vi "Text control 2 v2.8.vi"() -> ()   [LabVIEW 2016]
panel:
  in  "Set Start Time":dbl caption="Set Start Time (s)"
  out "Total lines":i32
  out "Line running":i32
  in  "byte count":u32=64
  in  "Serial Settings:Serial End Mode for Reads":u16(ring)=2 items=["None", "LastBit", "TermChar"]
  in  "Timeout (ms)":u32=10000
  in  "Enable Termination\nChar (T)":bool=TRUE
  in  "Termination char\n(0xA = '\\n' = LF)\n(0xD = '\\r' = CR)":u8=13 format="%.0x"
  in  "flow control":u16(ring) items=["None"=0, "XON/XOFF"=1, "RTS/CTS"=2, "DTR/DSR"=4]
  in  "stop bits":u16(ring)=10 items=["1.0"=10, "1.5"=15, "2.0"=20]
  in  "parity":u16(ring) items=["None", "Odd", "Even", "Mark", "Space"]
  in  "data bits":u16=8 min=5 max=8 step=1
  in  "VISA resource name":refnum<visa-resource-name>="COM6"
  in  "baud rate":u32=9600
  out "Serial port output":string
  out "error out":errorcluster
  in  "Units":bool
  out "Elapsed Time":dbl caption="Elapsed Time (s)"
  out "Id max vs time":cluster{"Y data in":dbl[], "X data in":dbl[]}[](graph)
  out "Ig":dbl format="%.2e"
  out "Id":dbl format="%.2e"
  out "Is":dbl format="%.2e"
  out "I vs Vg":cluster{"Y data in":dbl[], "X data in":dbl[]}[](graph)
  in  "Panel Controls 2":T1={"Emergency Stop"=refnum, "TransGraph Max"=1e-05, "Text/Graph (text=false)"=TRUE, "TransGraph Min"=1e-11} {"TransGraph Min" format="%.2e"; "TransGraph Max" format="%.2e"}
  out "Command running:":string="#output s 0 0 0 -0.008 0.008 0.002"
  in  "Standby":T2
  in  "Full Reset":bool
  in  "SMU4":cluster{"on/off":bool, "Voltage":dbl} {"Voltage" min=-100.0 max=100.0 format="%.2f"}
  in  "Source/Drain Range":u8(slide)=6 max=11 scale=0.0..11.0
  in  "Source/Drain\nRange mode":u16(ring) items=["Auto", "Limited", "Fixed"]
  in  "Gate Range":u8(slide)=6 max=11 scale=0.0..11.0
  in  "Gate Range\nmode":u16(ring) items=["Auto", "Limited", "Fixed"]
  in  "Gate":T3={"Gate Start"=0.0, "Gate Stop"=2.0, "Gate Step (linear only)"=1.0, "Gate Compliance"=0.0001, "Gate PComp"=0.0, "Range mode"=0, "Range"=6} {"Range" max=11 scale=0.0..11.0; "Range mode" items=["Auto", "Limited", "Fixed"]; "Gate PComp" format="%^.2e"; "Gate Compliance" format="%^.2e"; "Gate Step (linear only)" format="%^.4e"; "Gate Stop" format="%^.4e"; "Gate Start" format="%^.4e"}
  in  "Drain 2":T4={"Drain Start"=0.0, "Drain Stop"=2.0, "Drain Compliance"=0.0001, "Drain Step"=1.0, "Drain PComp"=0.0, "Range mode"=0, "Range"=6} {"Range" max=11 scale=0.0..11.0; "Range mode" items=["Auto", "Limited", "Fixed"]; "Drain PComp" format="%^.2e"; "Drain Step" format="%^.4e"; "Drain Compliance" format="%^.2e"; "Drain Stop" format="%^.4e"; "Drain Start" format="%^.4e"}
  in  "Timings 2":T5={"integration time"=0, "Short/Long integration time"=0.00064, "hold time (sec)"=0.0, "delay time (sec)"=0.0, "Step Time (0 disables)"=0.0, "sweep method"=0, "Pulse period"=0.005, "Base voltage"=0.0, "Pulse width"=0.0005} {"Pulse width" min=0.0005 max=0.1 step=0.0001 format="%.4f"; "Base voltage" format="%^.4e"; "Pulse period" min=0.005 max=1.0 step=0.0001 format="%.4f"; "sweep method" items=["Continuous", "Pulsed"]; "Step Time (0 disables)" format="%.2f"; "delay time (sec)" format="%.4f"; "hold time (sec)" format="%.4f"; "Short/Long integration time" format="%^.0e"; "integration time" scale=0.0..2.0}
  in  "Panel Controls":T6={"Emergency Stop"=refnum, "TransGraph Max"=1e-05, "Text/Graph (text=false)"=TRUE} {"TransGraph Max" format="%.2e"}
  in  "Interrupt run":bool
  in  "Drain: Compliance":dbl=0.001 format="%.8f"
  in  "Gate: Compliance":dbl=0.001 format="%.8f"
  out "Path":path=path "C:/users/rlp38/09Apr2009LTtesting/test2.txt"
  in  "hold time /s":dbl format="%.2f"
  in  "delay time /s":dbl format="%.2f"
  in  "integration time":u32(slide) max=2 step=1 scale=0.0..2.0
  in  "Integration time (short)":dbl=0.0019 min=8e-05 max=0.0019 step=8e-05 format="%^.0e"
  in  "Integration time (long)":dbl=0.32 min=0.04 max=2.0 step=0.02 format="%.2f"
  in  "Step delay /s":dbl format="%.2f"
  in  "Program":string="#pulsedstressV d 0.03 20 0 0.5 0.0827 5\n#\n#itime s\n#gaterangemode l\n#drainrangemode l\n#pulsed on 0.05 0 0.02\n#transfer d 1 -1 -0.1 -1 -1 0\n#wait-min 1\n#transfer d 1 -1 -0.1 -1 -1 0\n#output d 0 -1 -0.5 0 -1 -0.1\n#transfer d -10 40 1 5 40 35\n#transfer d -10 40 1 5 40 35\n#output d 0 40 20 0 40 1\n#\n#\n#sample 1 0.008 221 6 0.003\n#samplei 400e-6 200 6 0.002 0.1\n#vsu2pulse -10 4\n#\n#stressV 0.016 0.03 2e-4 0.1e-3 11\n#stressI 220e-7 0.08 15\n#transfer s -1 1 0.5 -0.005 0.005 0.005\n#output s 0 0 0 -0.008 0.008 0.002\n"
  # "Serial port settings"
  # "Time"
  # "Sec"
  # "Min"
  # "100 samples is approx 13s with medium integration"
  # "Syntax:\nitime [s|m|l]\ngaterangemode [a|l|f]\ndrainrangemode [a|l|f]\npulsed [on|off] PulsePeriod(sec) PulseBaseVoltage PulseONWidth(sec)\nstandby [on l off]\nwait NumMilliseconds\nwait-min NumMinutes\n# texthere = comment\ntransfer [s|d] VgStart VgStop VgStep VdStart VdStop VdStep\noutput [s|d] VgStart VgStop VgStep VdStart VdStop VdStep\nsample Vg Vd NumSamples Time(s) SampleInterval(s)\nsamplei Idg NumSamples Time(s) SampleInterval(s) VDGcompliance\n# if in doubt use SampleInterval(s) = 0.004\nstressV VG VD IGcompliance IDcompliance Duration(sec)\nstressI IDG VDGcompliance Duration(sec)\nvsu2pulse Bias Duration(s)\npulsedstressV [s|d] VEstop VgON VgOFF Period(s) PulseONwidth(s) Vd\nsample-fpp Vg Vd NumSamples Time\nresample-fpp Vg Vd\ntransfer-fpp [s|d] VgStart VgStop VgStep VdStart VdStop VdStep\noutput-fpp [s|d] VgStart VgStop VgStep VdStart VdStop VdStep\nserial SerialPortCommand"
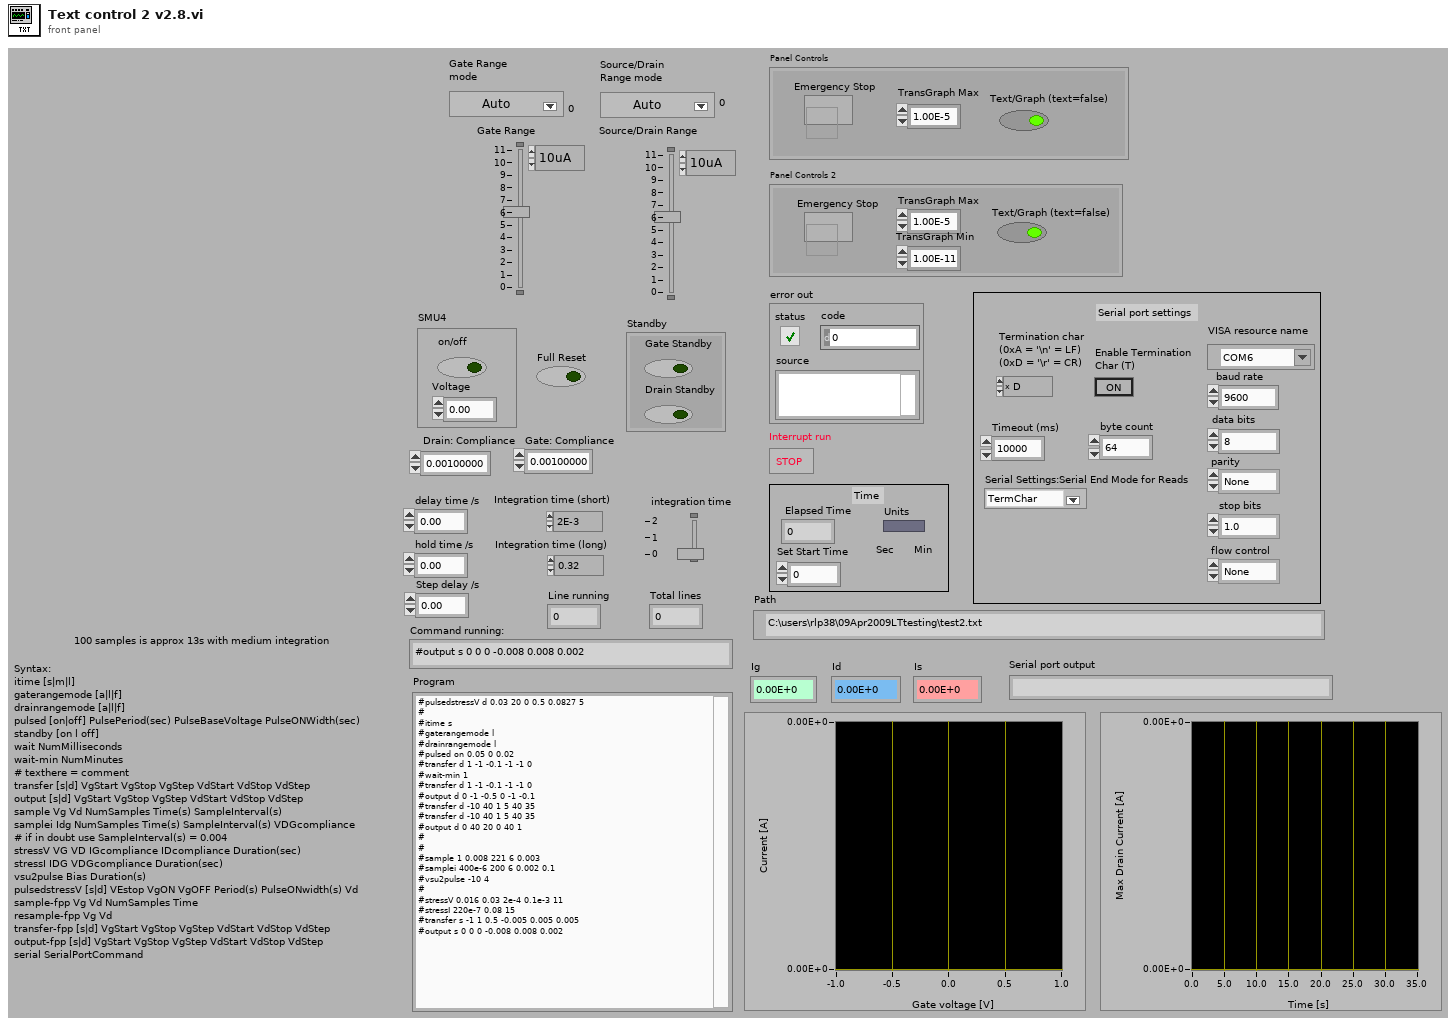
[diagram p1: front panel]
types:
  T1 = cluster{"Emergency Stop":refnum<vi>, "TransGraph Max":dbl, "Text/Graph (text=false)":bool, "TransGraph Min":dbl}
  T2 = cluster{"Gate Standby":bool, "Drain Standby":bool}
  T3 = cluster{"Gate Start":dbl, "Gate Stop":dbl, "Gate Step (linear only)":dbl, "Gate Compliance":dbl, "Gate PComp":dbl, "Range mode":u16, "Range":u8}
  T4 = cluster{"Drain Start":dbl, "Drain Stop":dbl, "Drain Compliance":dbl, "Drain Step":dbl, "Drain PComp":dbl, "Range mode":u16, "Range":u8}
  T5 = cluster{"integration time":u32, "Short/Long integration time":dbl, "hold time (sec)":dbl, "delay time (sec)":dbl, "Step Time (0 disables)":dbl, "sweep method":u16, "Pulse period":dbl, "Base voltage":dbl, "Pulse width":dbl}
  T6 = cluster{"Emergency Stop":refnum<vi>, "TransGraph Max":dbl, "Text/Graph (text=false)":bool}
  T7 = enum16{"open", "replace", "create", "open or create", "replace or create", "replace or create with confirmation"}
  T8 = cluster{"V2 Start":dbl, "V2 Step":dbl, "Number of points":i32}
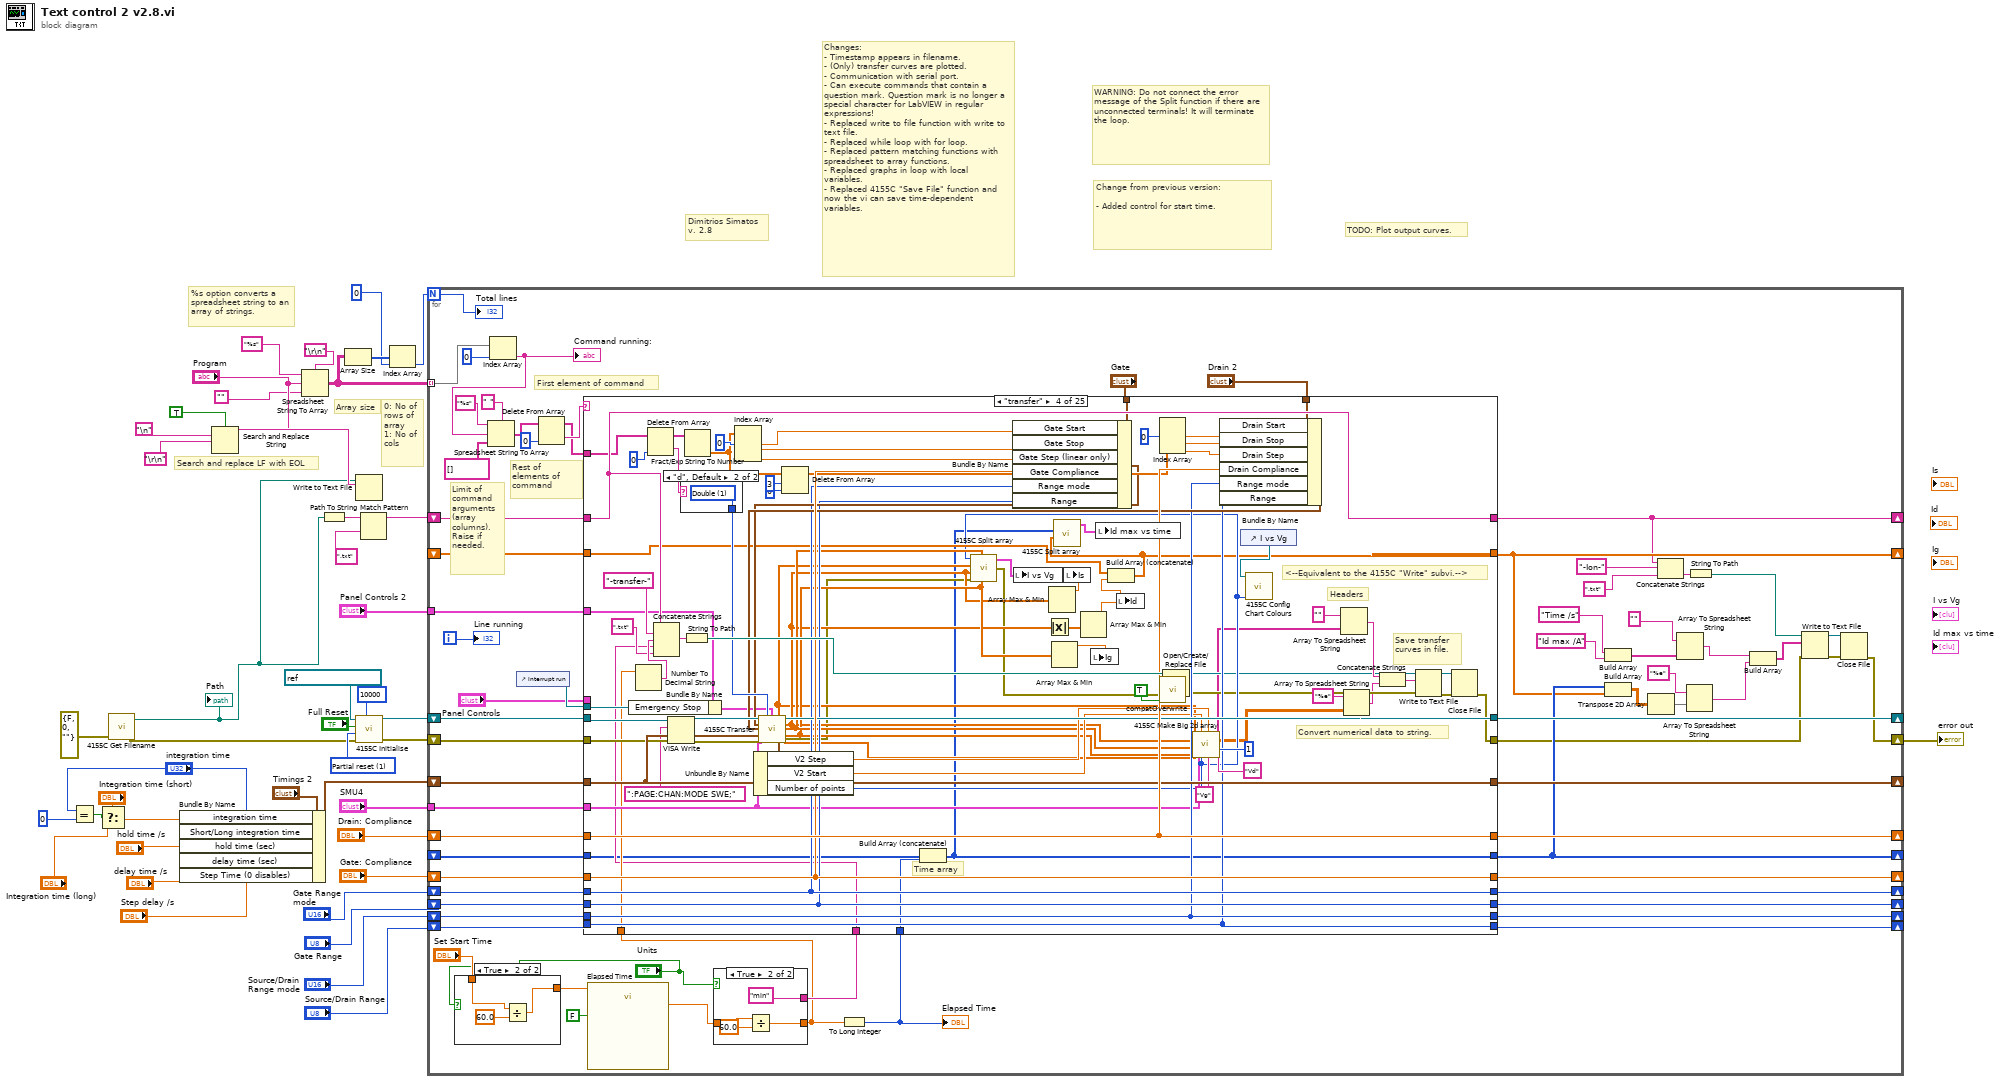
[diagram p0: block diagram]
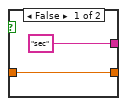
[diagram p3: hidden frame]
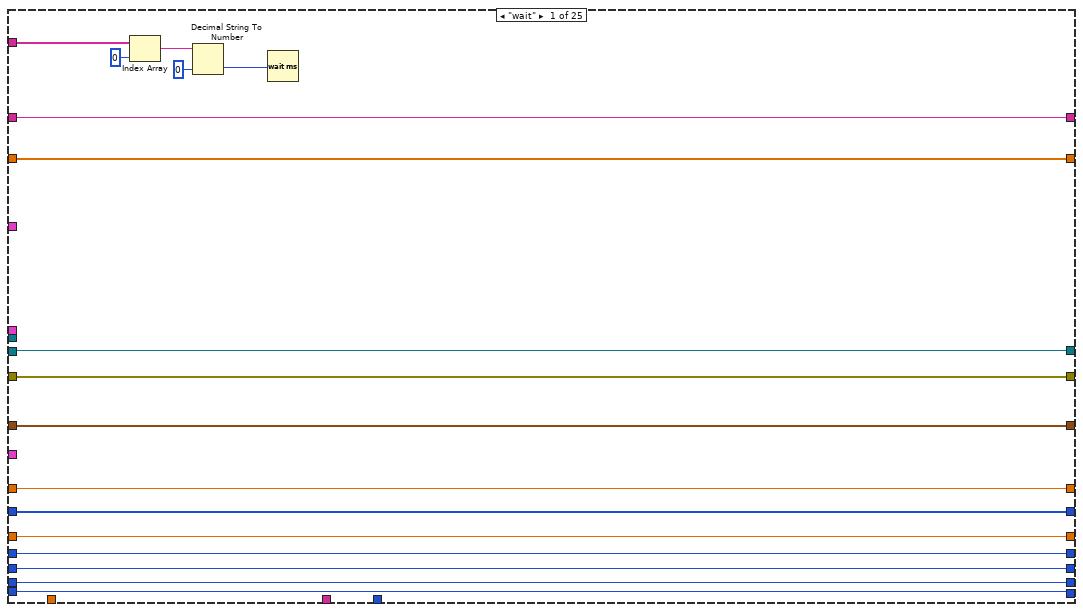
[diagram p4: hidden frame]
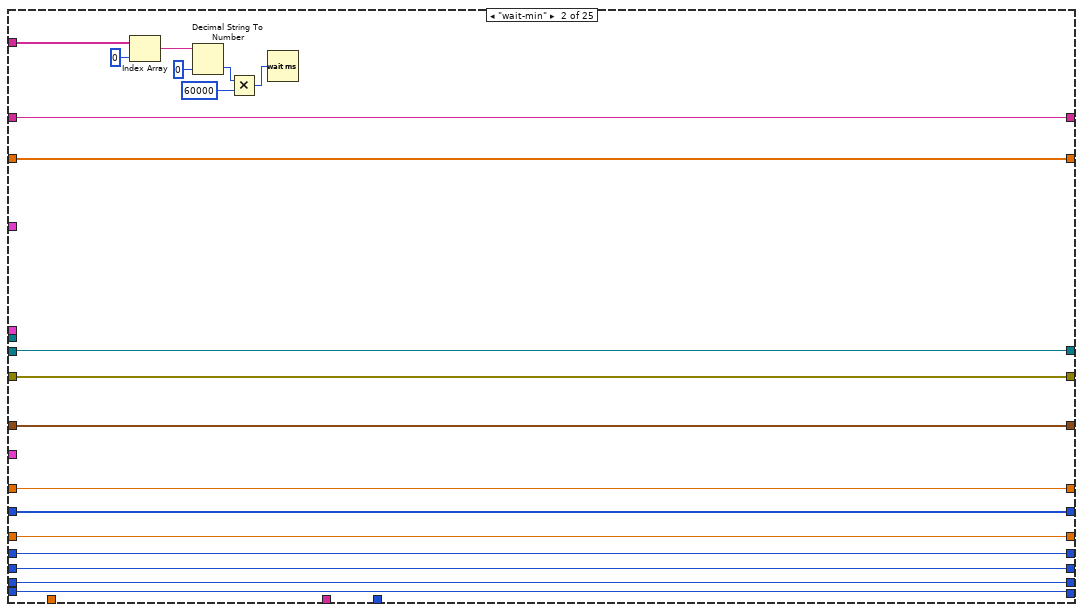
[diagram p5: hidden frame]
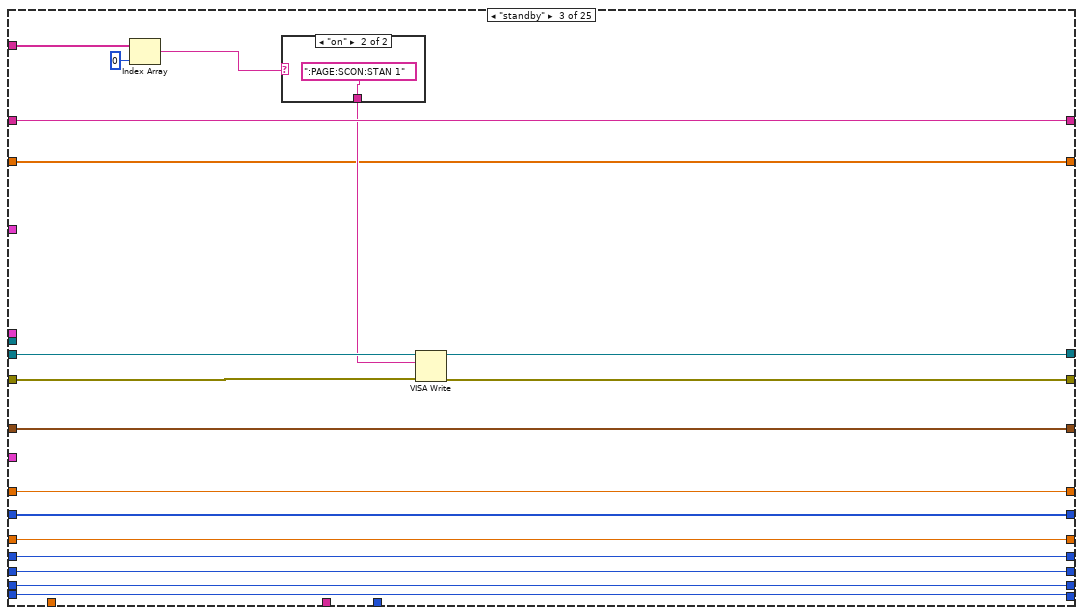
[diagram p6: hidden frame]
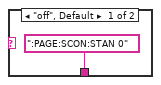
[diagram p7: hidden frame]
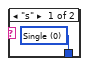
[diagram p8: hidden frame]
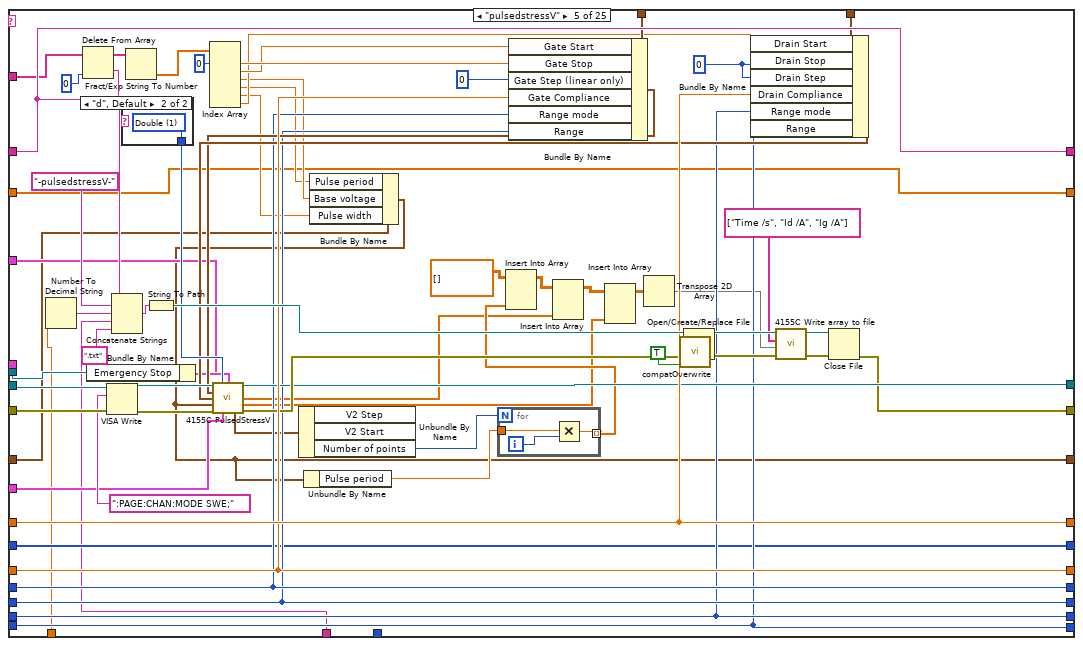
[diagram p9: hidden frame]
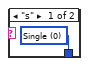
[diagram p10: hidden frame]
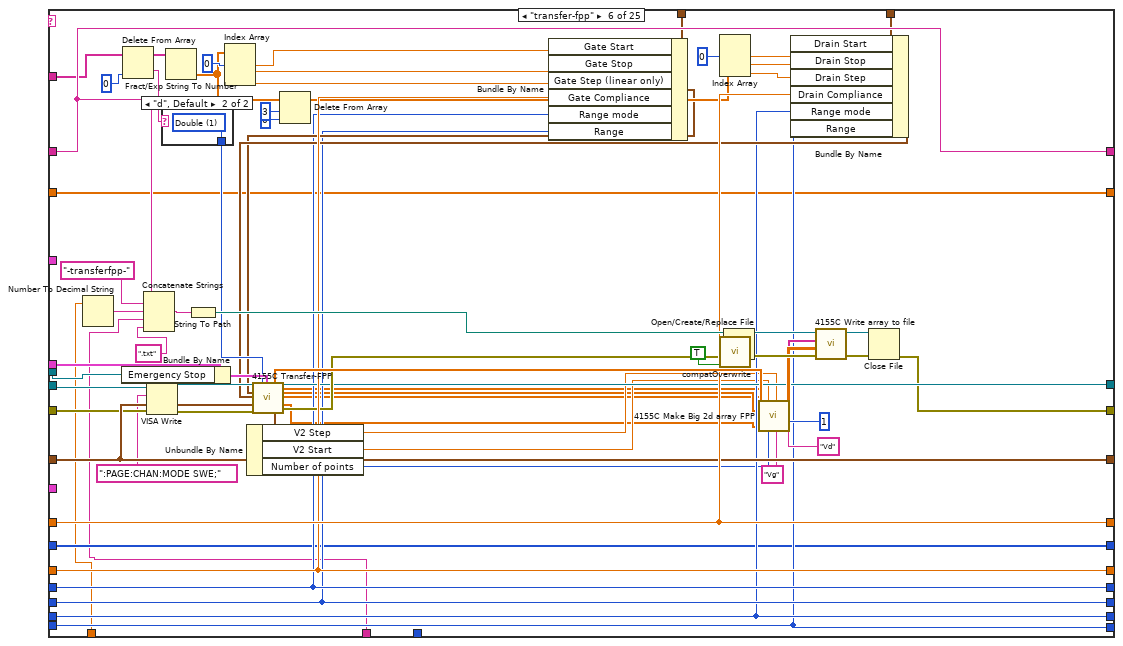
[diagram p11: hidden frame]
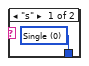
[diagram p12: hidden frame]
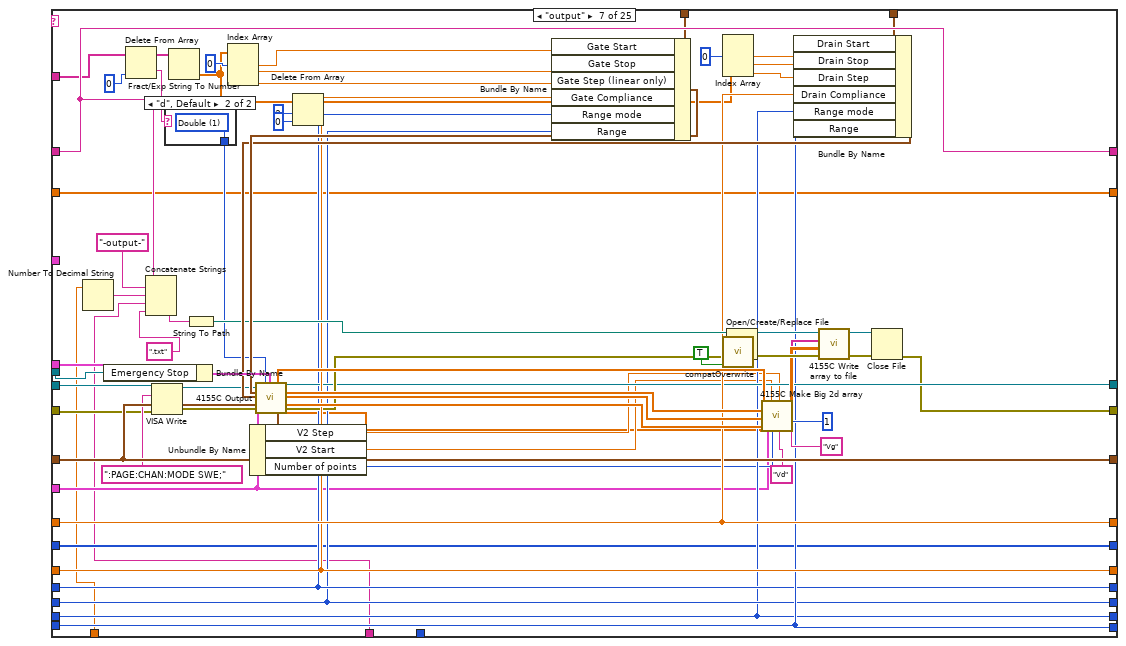
[diagram p13: hidden frame]
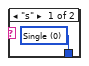
[diagram p14: hidden frame]
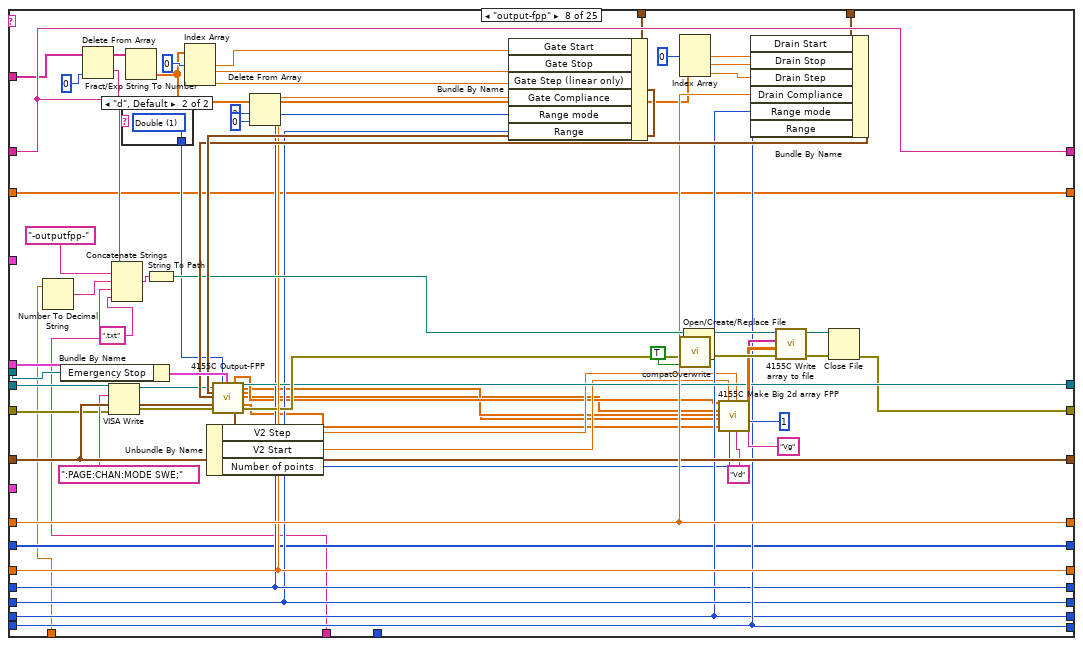
[diagram p15: hidden frame]
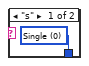
[diagram p16: hidden frame]
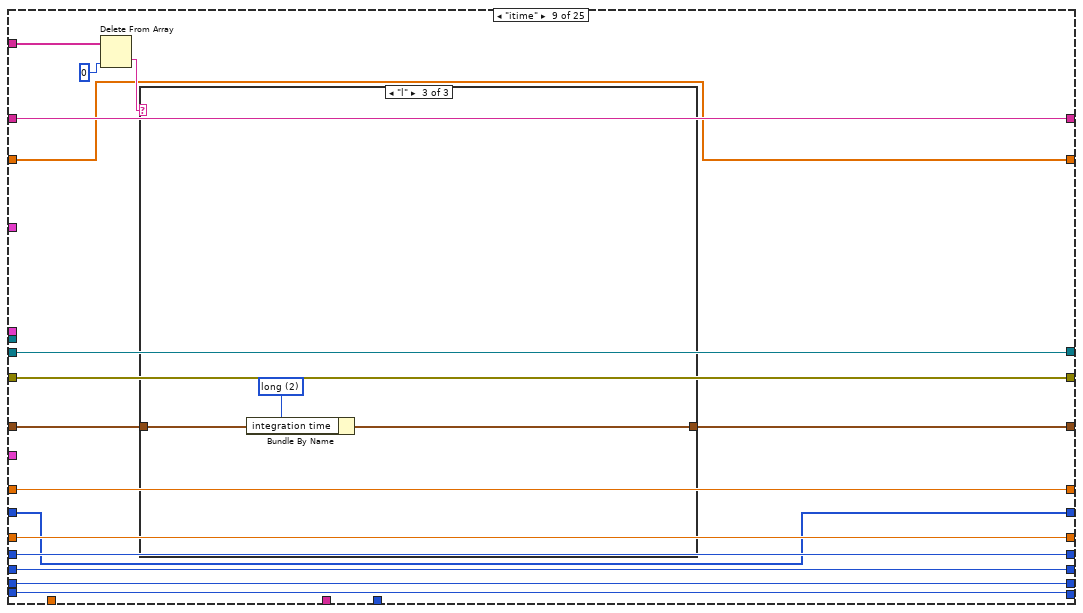
[diagram p17: hidden frame]
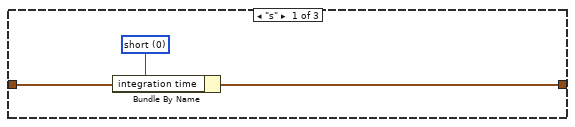
[diagram p18: hidden frame]
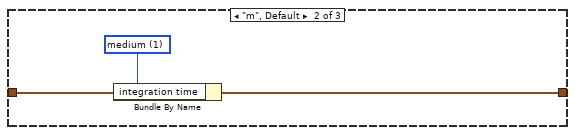
[diagram p19: hidden frame]
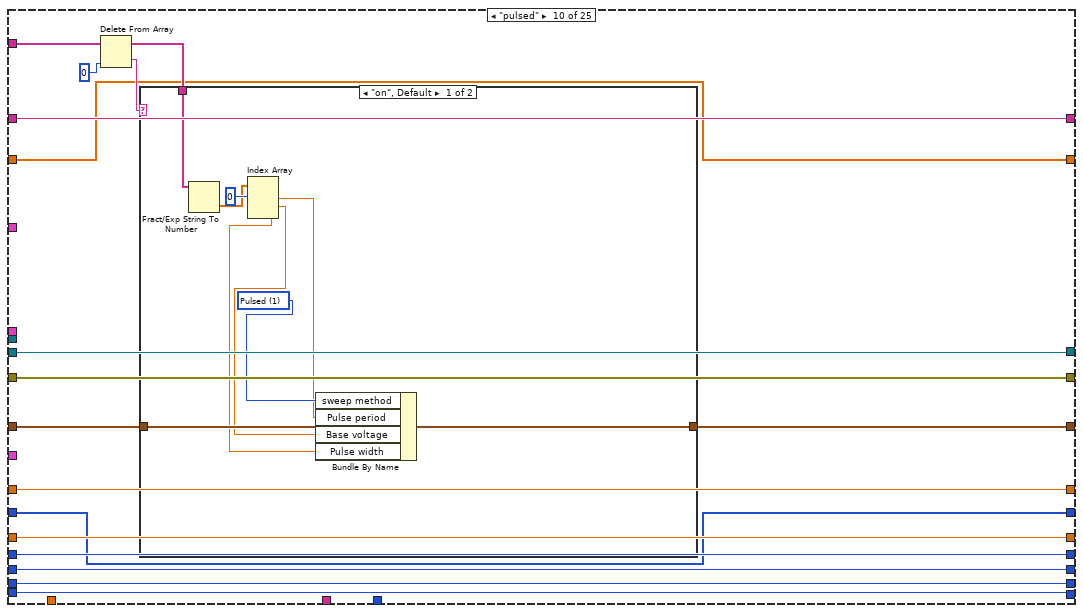
[diagram p20: hidden frame]
diagram:
  w35 = u16 1 items=["Reset All", "Partial reset"] ("Type of reset")
  # "TODO: Plot output curves."
  # "WARNING: Do not connect the error message of the Split function if there are unconnected terminals! It will terminate the loop."
  # "Array size"
  # "%s option converts a spreadsheet string to an array of strings."
  # "0: No of rows of array\n1: No of cols"
  # "Change from previous version:\n\n- Added control for start time."
  # "Dimitrios Simatos\nv. 2.8"
  # "Changes:\n- Timestamp appears in filename.\n- (Only) transfer curves are plotted.\n- Communication with serial port.\n- Can execute commands that contain a question mark. Question mark is no longer a special character for LabVIEW in regular expressions!\n- Replaced write to file function with write to text file.\n- Replaced while loop with for loop.\n- Replaced pattern matching functions with spreadsheet to array functions.\n- Replaced graphs in loop with local variables.\n- Replaced 4155C \"Save File\" function and now the vi can save time-dependent variables."
  # "Search and replace LF with EOL"
  n1 = Equal?(x="integration time", y=u32 0) -> (x = y?=w39:bool)
  n2 = Select(t="Integration time (short)", s=w39, f="Integration time (long)") -> (s? t:f=w43:dbl)
  n3 = call "4155C Get Filename.vi"("error in (no error)"=errorcluster {"status"=FALSE, "code"=0, "source"=""}) -> ("error out"=w30:errorcluster, "path"=w2:path)  [unwired: 2 in, 1 out]
  "Path" <- w2
  n4 = Bundle By Name(cluster="Timings 2", "integration time"="integration time", "Short/Long integration time"=w43, "hold time (sec)"="hold time /s", "delay time (sec)"="delay time /s", "Step Time (0 disables)"="Step delay /s") -> (w27:T5)
  n5 = Search and Replace String(replace all?=TRUE ("replace all? (F)"), input string="Program", search string="\n", replace string="\r\n") -> (result string=w17:string)  [unwired: 4 in, 3 out]
  n6 = Spreadsheet String To Array(delimiter (Tab)="\r\n", format string="%s", spreadsheet string="Program", array type (2D Dbl)="") -> (array=w8:string[][])
  n7 = Path To String(path=w2) -> (string=w5:string)
  n8 = Array Size(array=w8) -> (size(s)=w12:i32[])
  n9 = Write to Text File(file (use dialog)=w2, text=w17) -> ()  [unwired: 2 in, 3 out]
  n10 = call "4155C Initialise.vi"("VISA resource name in"=refnum<visa-resource-name> "GPIB0::14::INSTR", "Reset"="Full Reset", "Type of reset"=w35, "error in (no error)"=w30, "VISA Timeout Value"=u32 10000) -> ("VISA Resource Name out"=w29:refnum<visa-resource-name>, "error out"=w28:errorcluster)
  n11 = Match Pattern(string=w5, regular expression=".txt") -> (before substring=w3:string)  [unwired: 1 in, 3 out]
  n12 = Index Array(array=w12, index=0) -> (element=w10:i32)
  n13 = for {
    N: w10 -> [w77]
    tunnel: "SMU4" -> [w89]
    shift-left: "Source/Drain Range" -> [w94]
    shift-right: [w90] -> _
    shift-left: "Source/Drain\nRange mode" -> [w95]
    shift-right: [w91] -> _
    shift-left: "Gate Range" -> [w96]
    shift-right: [w92] -> _
    shift-left: "Gate Range\nmode" -> [w97]
    shift-right: [w93] -> _
    shift-left: "Gate: Compliance" -> [w106]
    shift-right: [w102] -> _
    shift-left: "Drain: Compliance" -> [w107]
    shift-right: [w103] -> _
    shift-left: w27 -> [w108]
    shift-right: [w104] -> _
    shift-left: w28 -> [w109]
    shift-right: [w45] -> w1
    shift-left: w29 -> [w110]
    shift-right: [w105] -> _
    shift-left: w3 -> [w111]
    shift-right: [w50] -> _
    tunnel: "Panel Controls 2" -> [w88]
    shift-right: [w53] -> _
    shift-left: _ -> [w87]
    shift-right: [w54] -> _
    shift-left: _ -> [w83]
    tunnel: w8 -> [w80] mode=indexing
    i -> [w78]
    # "Limit of command arguments (array columns). Raise if needed."
    # "Rest of elements of command"
    # "First element of command"
    n14 = case shown="True" "Units" {
      tunnel: "Set Start Time" -> [w112 w114]
      tunnel: [w112 w113] -> w48
      frame False {
      }
      frame True {
        n15 = Divide(x=w114, y=60.0) -> (x/y=w113:dbl)
      }
    }
    n16 = Index Array(array=w80, index=0 ("line index")) -> (element=w73:string)
    "Command running:" <- w73
    n17 = Spreadsheet String To Array(delimiter (Tab)=" ", format string="%s", spreadsheet string=w73, array type (2D Dbl)=string[] []) -> (array=w70:string[])
    n18 = control-ref of="Interrupt run"() -> (w101:refnum<vi>)
    n19 = Delete From Array(array=w70, index=0) -> (deleted portion=w71:string, array with subset deleted=w69:string[])  [unwired: 1 in]
    n20 = call "Elapsed Time"("Time Target (s)"=w48, "Auto Reset"=FALSE) -> ("Elapsed Time (s)"=w84:dbl)  [unwired: 10 in, 7 out]
    n21 = case shown="True" "Units" {
      tunnel: ["sec" "min"] -> w85
      tunnel: [w116 w120] -> w82
      tunnel: w84 -> [w116 w119]
      frame False {
      }
      frame True {
        n22 = Divide(x=w119, y=60.0) -> (x/y=w120:dbl)
      }
    }
    n23 = To Long Integer(number=w82) -> (32bit integer=w81:i32)
    "Elapsed Time" <- w81
    n24 = case shown="\"transfer\"" w71 {
      tunnel: w69 -> [w138 w157 w175 w252 w316 w385 w452 w527 w565 w591 w618 w643 w664 w678 _ _ w782 w843 _ w908 w952 w994 w1064 w1126 w1133]
      tunnel: w111 -> [w133 w153 w173 w259 w323 w393 w460 w535 w554 w580 w610 w636 w658 w671 w690 w732 w760 w825 w856 w895 w939 w982 w1058 w1122 w1135]
      tunnel: w110 -> [w132 w152 w164 w230 w307 w362 w428 w503 w555 w581 w611 w637 w659 w672 w695 w734 w788 w849 w860 w914 w958 w1000 w1070 w1080 w1139]
      tunnel: w109 -> [w131 w151 w163 w229 w306 w361 w425 w500 w556 w582 w612 w638 w660 w673 w694 w705 w787 w848 w859 w913 w957 w999 w1069 w1079 w1138]
      tunnel: w108 -> [w130 w150 w172 w255 w282 w389 w456 w531 w564 w590 w609 w635 w657 w670 w693 w729 w751 w817 w865 w888 w932 w975 w1057 w1121 w1140]
      tunnel: w107 -> [w129 w149 w171 w257 w321 w391 w458 w533 w563 w589 w617 w642 w663 w677 w692 w714 w786 w847 w868 w912 w956 w998 w1068 w1130 w1141]
      tunnel: w106 -> [w128 w148 w170 w256 w320 w390 w457 w532 w562 w588 w616 w641 w662 w676 w691 w715 w761 w826 w867 w896 w940 w983 w1059 w1123 w1143]
      tunnel: [w132 w152 w162 w254 w318 w387 w454 w529 w555 w581 w611 w637 w659 w672 w695 w734 w752 w799 w858 w889 w933 w976 w1010 w1082 w1139] -> w105
      tunnel: [w131 w151 w161 w253 w317 w386 w453 w528 w556 w582 w612 w638 w660 w673 w694 w704 w762 w800 w857 w897 w941 w984 w1009 w1081 w1137] -> w46
      tunnel: [w130 w150 w172 w255 w278 w389 w456 w531 w557 w583 w609 w635 w657 w670 w693 w729 w751 w817 w865 w888 w932 w975 w1057 w1121 w1140] -> w104
      tunnel: [w129 w149 w171 w257 w321 w391 w458 w533 w563 w589 w617 w642 w663 w677 w692 w714 w786 w847 w868 w912 w956 w998 w1068 w1130 w1141] -> w103
      tunnel: [w128 w148 w170 w256 w320 w390 w457 w532 w562 w588 w616 w641 w662 w676 w691 w715 w761 w826 w867 w896 w940 w983 w1059 w1123 w1143] -> w102
      tunnel: [w133 w153 w173 w259 w323 w393 w460 w535 w554 w580 w610 w636 w658 w671 w690 w732 w760 w825 w856 w895 w939 w982 w1058 w1122 w1135] -> w50
      tunnel: w101 -> [_ _ _ w262 w327 w398 w468 w539 _ _ _ _ _ _ _ _ w757 w822 _ w894 w938 w981 w1030 w1098 _]
      tunnel: "Gate" -> [_ _ _ w239 w310 w372 w439 w514 _ _ _ _ _ _ _ _ _ _ _ _ _ _ _ _ _]
      tunnel: "Drain 2" -> [_ _ _ w238 w309 w371 w438 w513 _ _ _ _ _ _ _ _ _ _ _ _ _ _ _ _ _]
      tunnel: "Panel Controls" -> [_ _ _ _ _ w370 w437 w512 _ _ _ _ _ _ _ _ _ _ _ _ _ _ _ _ _]
      tunnel: w97 -> [w127 w147 w169 w223 w300 w355 w423 w498 w561 w587 _ w634 w656 w669 w689 w716 w747 w813 w861 w884 w928 w971 w1053 w1117 w1144]
      tunnel: w96 -> [w126 w146 w168 w222 w299 w354 w422 w497 w560 w586 w615 _ w647 w675 w688 w717 w748 w814 w862 w885 w929 w972 w1054 w1118 w1145]
      tunnel: w95 -> [w125 w145 w167 w221 w298 w353 w421 w496 w559 w585 w614 w640 w661 _ w687 w718 w749 w815 w863 w886 w930 w973 w1055 w1119 w1146]
      tunnel: w94 -> [w124 w144 w166 w220 w297 w352 w424 w499 w558 w584 w613 w639 _ w674 w686 w719 w750 w816 w864 w887 w931 w974 w1056 w1120 w1147]
      tunnel: [w127 w147 w169 w223 w300 w355 w423 w498 w561 w587 w608 w634 w656 w669 w689 w716 w747 w813 w861 w884 w928 w971 w1053 w1117 w1144] -> w93
      tunnel: [w126 w146 w168 w222 w299 w354 w422 w497 w560 w586 w615 w626 w647 w675 w688 w717 w748 w814 w862 w885 w929 w972 w1054 w1118 w1145] -> w92
      tunnel: [w125 w145 w167 w221 w298 w353 w421 w496 w559 w585 w614 w640 w661 w668 w687 w718 w749 w815 w863 w886 w930 w973 w1055 w1119 w1146] -> w91
      tunnel: [w124 w144 w166 w220 w297 w352 w424 w499 w558 w584 w613 w639 w648 w674 w686 w719 w750 w816 w864 w887 w931 w974 w1056 w1120 w1147] -> w90
      tunnel: w89 -> [_ _ _ w215 w294 _ w416 _ _ _ _ _ _ _ _ _ _ _ _ _ _ _ _ _ _]
      tunnel: w88 -> [_ _ _ w213 w293 _ _ _ _ _ _ _ _ _ _ _ _ _ _ _ _ _ _ _ _]
      tunnel: [w123 w140 w159 w181 w270 w342 w413 w485 w553 w578 w607 w625 w646 w667 w685 w700 w739 w797 w855 w873 w921 w965 w1007 w1075 w1136] -> w53
      tunnel: w87 -> [w123 w140 w159 w204 w270 w342 w413 w485 w553 w578 w607 w625 w646 w667 w685 w700 w739 w797 w855 w873 w921 w965 w1007 w1075 w1136]
      tunnel: w82 -> [_ _ _ w200 w267 w340 w410 w482 _ _ _ _ _ _ _ w698 w737 w794 _ w870 w918 w962 w1004 w1071 _]
      tunnel: w85 -> [_ _ _ w197 w266 w338 w409 w481 _ _ _ _ _ _ _ w696 w735 w793 _ w869 w917 w961 w1003 w1072 _]
      tunnel: w81 -> [_ _ _ w182 _ _ _ _ _ _ _ _ _ _ _ _ _ _ _ _ _ _ _ _ _]
      tunnel: [w122 w139 w158 w180 w269 w341 w412 w484 w552 w577 w606 w624 w645 w666 w684 w699 w738 w796 w854 w872 w920 w964 w1006 w1074 w1142] -> w54
      tunnel: w83 -> [w122 w139 w158 w196 w269 w341 w412 w484 w552 w577 w606 w624 w645 w666 w684 w699 w738 w796 w854 w872 w920 w964 w1006 w1074 w1142]
      frame "wait" {
        n25 = Index Array(array=w138, index=0 ("Index")) -> (element=w136:string)
        n26 = Decimal String To Number(string=w136, default (0L)=u32 0) -> (number=w135:u32)  [unwired: 1 in, 1 out]
        n27 = Wait (ms)(milliseconds to wait=w135) -> ()  [unwired: 1 out]
      }
      frame "wait-min" {
        n28 = Index Array(array=w157, index=0 ("Index")) -> (element=w155:string)
        n29 = Decimal String To Number(string=w155, default (0L)=u32 0) -> (number=w143:u32)  [unwired: 1 in, 1 out]
        n30 = Multiply(x=w143, y=u32 60000) -> (x*y=w142:u32)
        n31 = Wait (ms)(milliseconds to wait=w142) -> ()  [unwired: 1 out]
      }
      frame "standby" {
        n32 = Index Array(array=w175, index=0 ("Index")) -> (element=w165:string)
        n33 = case shown="\"on\"" w165 {
          tunnel: [":PAGE:SCON:STAN 0" ":PAGE:SCON:STAN 1"] -> w160
          frame "off", Default {
          }
          frame "on" {
          }
        }
        n34 = VISA Write(VISA resource name=w164, write buffer=w160, error in (no error)=w163) -> (VISA resource name out=w162:refnum<visa-resource-name>, error out=w161:errorcluster)  [unwired: 1 out]
      }
      frame "transfer" {
        # "<--Equivalent to the 4155C \"Write\" subvi.-->"
        # "Headers"
        # "Convert numerical data to string."
        # "Save transfer curves in file."
        # "Time array"
        n35 = Bundle By Name(cluster=w213, "Emergency Stop"=w262) -> (w214:T1)
        n36 = Number To Decimal String(number=w200) -> (decimal integer string=w199:string)  [unwired: 1 in]
        n37 = Delete From Array(array=w252, index=0 ("Index")) -> (deleted portion=w250:string, array with subset deleted=w249:string[])  [unwired: 1 in]
        n38 = Concatenate Strings(w259, "-transfer-" ("Prefix"), w199, w197, ".txt" ("Suffix")) -> (w261:string)
        n39 = VISA Write(VISA resource name=w230, write buffer=":PAGE:CHAN:MODE SWE;" ("write buffer (\"\")"), error in (no error)=w229) -> (VISA resource name out=w227:refnum<visa-resource-name>, error out=w228:errorcluster)  [unwired: 1 out]
        n40 = case shown="\"d\", Default" w250 {
          tunnel: [w264 w265] -> w248
          frame "s" {
            w264 = u16 0 items=["Single", "Double"] ("sweep mode")
          }
          frame "d", Default {
            w265 = u16 1 items=["Single", "Double"] ("sweep mode")
          }
        }
        n41 = String To Path(string=w261) -> (path=w258:path)
        n42 = Fract/Exp String To Number(string=w249) -> (number=w234:dbl[])  [unwired: 3 in, 1 out]
        n43 = Index Array(array=w234, index #1=0 ("Index")) -> (element #1=w247:dbl, element #2=w246:dbl, element #3=w245:dbl)  [unwired: 2 in]
        n44 = Delete From Array(array=w234, length=3 ("Length"), index=0 ("Index")) -> (array with subset deleted=w232:dbl[])  [unwired: 1 out]
        n45 = Build Array (concatenate)(w196, w182) -> (w180:i32[])
        n46 = Bundle By Name(cluster=w239, "Gate Start"=w247, "Gate Stop"=w246, "Gate Step (linear only)"=w245, "Gate Compliance"=w256, "Range mode"=w223, "Range"=w222) -> (w224:T3)
        n47 = Index Array(array=w232, index #1=0 ("Index")) -> (element #1=w242:dbl, element #2=w241:dbl, element #3=w240:dbl)  [unwired: 2 in]
        n48 = call <vilib>:"compatOverwrite.vi"("overwrite (F)"=TRUE) -> ("overwrite?"=w212:T7)
        n49 = Bundle By Name(cluster=w238, "Drain Start"=w242, "Drain Stop"=w241, "Drain Step"=w240, "Drain Compliance"=w257, "Range mode"=w221, "Range"=w220) -> (w225:T4)
        n50 = call "4155C Transfer.vi"("VISA resource name in"=w227, "Gate"=w224, "Drain"=w225, "Timings"=w255, "error in (no error)"=w228, "SMU4"=w215, "sweep mode"=w248, "Panel Controls"=w214) -> ("VG"=w205:dbl[], "Outparams"=w219:T8, "VISA Resource Name out"=w254:refnum<visa-resource-name>, "IS"=w206:dbl[], "ID"=w211:dbl[], "IG"=w207:dbl[], "error out"=w192:errorcluster, "SMU4"=w216:dbl[])  [unwired: 12 in]
        n51 = Unbundle By Name(w219) -> ("V2 Step"=w218:dbl, "V2 Start"=w217:dbl, "Number of points"=w202:i32)
        n52 = call "4155C Split array.vi"("Number of VAR2 steps"=w202, "Y2 data in"=w211, "X data in"=w205, "Y1 data in"=w206, "Y3 data in"=w207, "error in (no error)"=w192) -> ("Array of clusters"=w195:cluster{"Y data in":dbl[], "X data in":dbl[]}[], "error out"=w193:errorcluster)  [unwired: 1 in]
        n53 = local write "I vs Vg"(w195) -> ()
        n54 = Absolute Value(x=w206) -> (abs(x)=w210:dbl[])
        n55 = Array Max & Min(array=w206) -> (max value=w208:dbl)  [unwired: 3 out]
        n56 = Array Max & Min(array=w207) -> (max value=w209:dbl)  [unwired: 3 out]
        n57 = local write "Is"(w208) -> ()
        n58 = Array Max & Min(array=w210) -> (max value=w203:dbl)  [unwired: 3 out]
        n59 = local write "Ig"(w209) -> ()
        n60 = Build Array (concatenate)(w204, w203) -> (w181:dbl[])
        n61 = call "4155C Split array.vi"("X data in"=w180, "Y1 data in"=w181) -> ("Array of clusters"=w194:cluster{"Y data in":dbl[], "X data in":dbl[]}[])  [unwired: 5 in, 1 out]
        n62 = local write "Id max vs time"(w194) -> ()
        n63 = local write "Id"(w203) -> ()
        n64 = Open/Create/Replace File(file path (use dialog)=w258, error in=w193, operation (0:open)=w212) -> (refnum out=w179:refnum<file>, error out=w189:errorcluster)  [unwired: 3 in, 1 out]
        n65 = call "4155C Make Big 2d array.vi"("1D Var1"=w205, "1d IS"=w206, "1d ID"=w211, "1d IG"=w207, "1d SMU4"=w216, "SMU4"=w215, "VAR2 START"=w217, "Number of VAR2 steps"=w202, "VAR2 STEP"=w218, "VAR1 Name"="Vg", "Decimal places in header"=i8 1, "VAR2 Name"="Vd") -> ("Header array"=w178:string[], "Data array"=w186:dbl[][])  [unwired: 14 in]
        n66 = control-ref of="I vs Vg"() -> (w201:refnum<vi>)
        n67 = call "4155C Config Chart Colours.vi"("Numeric"=w202, "XY Graph 2"=w201) -> ()  [unwired: 6 in]
        n68 = Array To Spreadsheet String(array=w178, 3:"" ("format string")) -> (spreadsheet string=w185:string)  [unwired: 1 in]
        n69 = Array To Spreadsheet String(array=w186, 3:"%e" ("format string")) -> (spreadsheet string=w188:string)  [unwired: 1 in]
        n70 = Concatenate Strings(w185, w188) -> (w187:string)
        n71 = Write to Text File(file (use dialog)=w179, text=w187, error in=w189) -> (refnum out=w191:refnum<file>, error out=w190:errorcluster)  [unwired: 1 in, 1 out]
        n72 = Close File(refnum=w191, error in=w190) -> (error out=w253:errorcluster)  [unwired: 1 out]
      }
      frame "pulsedstressV" {
        w276 = 0
        n73 = Number To Decimal String(number=w267) -> (decimal integer string=w324:string)  [unwired: 1 in]
        n74 = Delete From Array(array=w316, index=0 ("Index")) -> (deleted portion=w314:string, array with subset deleted=w313:string[])  [unwired: 1 in]
        n75 = Bundle By Name(cluster=w293, "Emergency Stop"=w327) -> (w295:T1)
        n76 = VISA Write(VISA resource name=w307, write buffer=":PAGE:CHAN:MODE SWE;" ("write buffer (\"\")"), error in (no error)=w306) -> (VISA resource name out=w304:refnum<visa-resource-name>, error out=w305:errorcluster)  [unwired: 1 out]
        n77 = Concatenate Strings(w323, "-pulsedstressV-" ("Substring"), w324, w266, ".txt" ("Substring")) -> (w326:string)
        n78 = case shown="\"d\", Default" w314 {
          tunnel: [w336 w337] -> w312
          frame "s" {
            w336 = u16 0 items=["Single", "Double"] ("sweep mode")
          }
          frame "d", Default {
            w337 = u16 1 items=["Single", "Double"] ("sweep mode")
          }
        }
        n79 = Fract/Exp String To Number(string=w313) -> (number=w308:dbl[])  [unwired: 3 in, 1 out]
        n80 = String To Path(string=w326) -> (path=w322:path)
        n81 = Index Array(array=w308, index #1=0 ("Index")) -> (element #1=w285:dbl, element #2=w284:dbl, element #3=w281:dbl, element #4=w280:dbl, element #5=w279:dbl, element #6=w283:dbl)  [unwired: 5 in]
        n82 = Bundle By Name(cluster=w282, "Pulse period"=w280, "Base voltage"=w281, "Pulse width"=w279) -> (w278:T5)
        n83 = Unbundle By Name(w278) -> ("Pulse period"=w286:dbl)
        n84 = Bundle By Name(cluster=w310, "Gate Start"=w284, "Gate Stop"=w285, "Gate Step (linear only)"=0, "Gate Compliance"=w320, "Range mode"=w300, "Range"=w299) -> (w301:T3)
        n85 = call <vilib>:"compatOverwrite.vi"("overwrite (F)"=TRUE) -> ("overwrite?"=w271:T7)
        n86 = Bundle By Name(cluster=w309, "Drain Start"=w283, "Drain Stop"=w276, "Drain Step"=w276, "Drain Compliance"=w321, "Range mode"=w298, "Range"=w297) -> (w302:T4)
        n87 = call "4155C PulsedStressV.vi"("VISA resource name in"=w304, "sweep mode"=w312, "Panel Controls"=w295, "Gate"=w301, "Drain"=w302, "Timings"=w278, "error in (no error)"=w305, "SMU4"=w294) -> ("VISA Resource Name out"=w318:refnum<visa-resource-name>, "ID"=w274:dbl[], "IG"=w272:dbl[], "Outparams"=w296:T8, "error out"=w319:errorcluster)  [unwired: 3 in]
        n88 = Unbundle By Name(w296) -> ("Number of points"=w273:i32)  [unwired: 2 out]
        n89 = for {
          N: w273 -> [_]
          tunnel: [w333] -> w275 mode=indexing
          tunnel: w286 -> [w335]
          i -> [w334]
          n90 = Multiply(x=w335, y=w334) -> (x*y=w333:dbl)
        }
        n91 = Insert Into Array(array=dbl[][] [] ("Input Array"), new element=w275) -> (w287:dbl[][])  [unwired: 2 in]
        n92 = Insert Into Array(array=w287, new element=w274) -> (w292:dbl[][])  [unwired: 2 in]
        n93 = Insert Into Array(array=w292, new element=w272) -> (w291:dbl[][])  [unwired: 2 in]
        n94 = Transpose 2D Array(2D array=w291) -> (transposed array=w290:dbl[][])
        n95 = Open/Create/Replace File(file path (use dialog)=w322, error in=w319, operation (0:open)=w271) -> (refnum out=w330:refnum<file>, error out=w331:errorcluster)  [unwired: 3 in, 1 out]
        n96 = call "4155C Write array to file.vi"("Byte Stream File Refnum"=w330, "Header"=string[] ["Time /s", "Id /A", "Ig /A"], "Data Array"=w290, "error in (no error)"=w331) -> ("dup refnum"=w328:refnum<file>, "error out"=w329:errorcluster)  [unwired: 1 in]
        n97 = Close File(refnum=w328, error in=w329) -> (error out=w317:errorcluster)  [unwired: 1 out]
      }
      frame "transfer-fpp" {
        n98 = Number To Decimal String(number=w340) -> (decimal integer string=w394:string)  [unwired: 1 in]
        n99 = Bundle By Name(cluster=w370, "Emergency Stop"=w398) -> (w406:T6)
        n100 = Delete From Array(array=w385, index=0 ("Index")) -> (deleted portion=w383:string, array with subset deleted=w382:string[])  [unwired: 1 in]
        n101 = Concatenate Strings(w393, "-transferfpp-" ("Substring"), w394, w338, ".txt" ("Substring")) -> (w396:string)
        n102 = VISA Write(VISA resource name=w362, write buffer=":PAGE:CHAN:MODE SWE;" ("write buffer (\"\")"), error in (no error)=w361) -> (VISA resource name out=w359:refnum<visa-resource-name>, error out=w360:errorcluster)  [unwired: 1 out]
        n103 = case shown="\"d\", Default" w383 {
          tunnel: [w407 w408] -> w381
          frame "s" {
            w407 = u16 0 items=["Single", "Double"] ("sweep mode")
          }
          frame "d", Default {
            w408 = u16 1 items=["Single", "Double"] ("sweep mode")
          }
        }
        n104 = Fract/Exp String To Number(string=w382) -> (number=w366:dbl[])  [unwired: 3 in, 1 out]
        n105 = String To Path(string=w396) -> (path=w392:path)
        n106 = Index Array(array=w366, index #1=0 ("Index")) -> (element #1=w380:dbl, element #2=w379:dbl, element #3=w378:dbl)  [unwired: 2 in]
        n107 = Delete From Array(array=w366, length=3 ("Length"), index=0 ("Index")) -> (array with subset deleted=w364:dbl[])  [unwired: 1 out]
        n108 = Bundle By Name(cluster=w372, "Gate Start"=w380, "Gate Stop"=w379, "Gate Step (linear only)"=w378, "Gate Compliance"=w390, "Range mode"=w355, "Range"=w354) -> (w356:T3)
        n109 = Index Array(array=w364, index #1=0 ("Index")) -> (element #1=w375:dbl, element #2=w374:dbl, element #3=w373:dbl)  [unwired: 2 in]
        n110 = call <vilib>:"compatOverwrite.vi"("overwrite (F)"=TRUE) -> ("overwrite?"=w343:T7)
        n111 = Bundle By Name(cluster=w371, "Drain Start"=w375, "Drain Stop"=w374, "Drain Step"=w373, "Drain Compliance"=w391, "Range mode"=w353, "Range"=w352) -> (w357:T4)
        n112 = call "4155C Transfer-FPP.vi"("VISA resource name in"=w359, "Gate"=w356, "Drain"=w357, "Timings"=w389, "error in (no error)"=w360, "sweep mode"=w381, "Panel Controls"=w406) -> ("VG"=w397:dbl[], "Outparams"=w351:T8, "VISA Resource Name out"=w387:refnum<visa-resource-name>, "Vprobe2"=w347:dbl[], "ID"=w346:dbl[], "IG"=w345:dbl[], "Vprobe1"=w344:dbl[], "error out"=w388:errorcluster)  [unwired: 13 in]
        n113 = Unbundle By Name(w351) -> ("V2 Step"=w350:dbl, "V2 Start"=w349:dbl, "Number of points"=w348:i32)
        n114 = Open/Create/Replace File(file path (use dialog)=w392, error in=w388, operation (0:open)=w343) -> (refnum out=w403:refnum<file>, error out=w404:errorcluster)  [unwired: 3 in, 1 out]
        n115 = call "4155C Make Big 2d array FPP.vi"("1D Var1"=w397, "1d ID"=w346, "1d Vp2"=w347, "1d IG"=w345, "1d Vp1"=w344, "VAR2 START"=w349, "Number of VAR2 steps"=w348, "VAR2 STEP"=w350, "VAR1 Name"="Vg", "Decimal places in header"=i8 1, "VAR2 Name"="Vd") -> ("Header array"=w399:string[], "Data array"=w400:dbl[][])  [unwired: 15 in]
        n116 = call "4155C Write array to file.vi"("Byte Stream File Refnum"=w403, "Header"=w399, "Data Array"=w400, "error in (no error)"=w404) -> ("dup refnum"=w401:refnum<file>, "error out"=w402:errorcluster)  [unwired: 1 in]
        n117 = Close File(refnum=w401, error in=w402) -> (error out=w386:errorcluster)  [unwired: 1 out]
      }
      frame "output" {
        n118 = Number To Decimal String(number=w410) -> (decimal integer string=w461:string)  [unwired: 1 in]
        n119 = Bundle By Name(cluster=w437, "Emergency Stop"=w468) -> (w478:T6)
        n120 = Delete From Array(array=w452, index=0 ("Index")) -> (deleted portion=w450:string, array with subset deleted=w449:string[])  [unwired: 1 in]
        n121 = Concatenate Strings(w460, "-output-" ("Substring"), w461, w409, ".txt" ("Substring")) -> (w463:string)
        n122 = VISA Write(VISA resource name=w428, write buffer=":PAGE:CHAN:MODE SWE;" ("write buffer (\"\")"), error in (no error)=w425) -> (VISA resource name out=w427:refnum<visa-resource-name>, error out=w426:errorcluster)  [unwired: 1 out]
        n123 = case shown="\"d\", Default" w450 {
          tunnel: [w479 w480] -> w448
          frame "s" {
            w479 = u16 0 items=["Single", "Double"] ("sweep mode")
          }
          frame "d", Default {
            w480 = u16 1 items=["Single", "Double"] ("sweep mode")
          }
        }
        n124 = Fract/Exp String To Number(string=w449) -> (number=w431:dbl[])  [unwired: 3 in, 1 out]
        n125 = String To Path(string=w463) -> (path=w459:path)
        n126 = Index Array(array=w431, index #1=0 ("Index")) -> (element #1=w447:dbl, element #2=w446:dbl, element #3=w445:dbl)  [unwired: 2 in]
        n127 = Delete From Array(array=w431, length=3 ("Length"), index=0 ("Index")) -> (array with subset deleted=w430:dbl[])  [unwired: 1 out]
        n128 = Bundle By Name(cluster=w439, "Gate Start"=w447, "Gate Stop"=w446, "Gate Step (linear only)"=w445, "Gate Compliance"=w457, "Range mode"=w423, "Range"=w422) -> (w477:T3)
        n129 = Index Array(array=w430, index #1=0 ("Index")) -> (element #1=w442:dbl, element #2=w441:dbl, element #3=w440:dbl)  [unwired: 2 in]
        n130 = call <vilib>:"compatOverwrite.vi"("overwrite (F)"=TRUE) -> ("overwrite?"=w414:T7)
        n131 = Bundle By Name(cluster=w438, "Drain Start"=w442, "Drain Stop"=w441, "Drain Step"=w440, "Drain Compliance"=w458, "Range mode"=w421, "Range"=w424) -> (w476:T4)
        n132 = call "4155C Output.vi"("VISA resource name in"=w427, "Gate"=w477, "Drain"=w476, "Timings"=w456, "error in (no error)"=w426, "SMU4"=w416, "sweep mode"=w448, "Panel controls"=w478) -> ("VD"=w464:dbl[], "Outparams"=w419:T8, "VISA Resource Name out"=w454:refnum<visa-resource-name>, "IS"=w467:dbl[], "ID"=w466:dbl[], "IG"=w465:dbl[], "error out"=w455:errorcluster, "SMU4"=w415:dbl[])  [unwired: 12 in]
        n133 = Unbundle By Name(w419) -> ("V2 Step"=w420:dbl, "V2 Start"=w418:dbl, "Number of points"=w417:i32)
        n134 = Open/Create/Replace File(file path (use dialog)=w459, error in=w455, operation (0:open)=w414) -> (refnum out=w473:refnum<file>, error out=w474:errorcluster)  [unwired: 3 in, 1 out]
        n135 = call "4155C Make Big 2d array.vi"("1D Var1"=w464, "1d IS"=w467, "1d ID"=w466, "1d IG"=w465, "1d SMU4"=w415, "SMU4"=w416, "VAR2 START"=w418, "Number of VAR2 steps"=w417, "VAR2 STEP"=w420, "VAR1 Name"="Vd", "Decimal places in header"=i8 1, "VAR2 Name"="Vg") -> ("Header array"=w469:string[], "Data array"=w470:dbl[][])  [unwired: 14 in]
        n136 = call "4155C Write array to file.vi"("Byte Stream File Refnum"=w473, "Header"=w469, "Data Array"=w470, "error in (no error)"=w474) -> ("dup refnum"=w471:refnum<file>, "error out"=w472:errorcluster)  [unwired: 1 in]
        n137 = Close File(refnum=w471, error in=w472) -> (error out=w453:errorcluster)  [unwired: 1 out]
      }
      frame "output-fpp" {
        n138 = Number To Decimal String(number=w482) -> (decimal integer string=w536:string)  [unwired: 1 in]
        n139 = Bundle By Name(cluster=w512, "Emergency Stop"=w539) -> (w549:T6)
        n140 = Delete From Array(array=w527, index=0 ("Index")) -> (deleted portion=w525:string, array with subset deleted=w524:string[])  [unwired: 1 in]
        n141 = VISA Write(VISA resource name=w503, write buffer=":PAGE:CHAN:MODE SWE;" ("write buffer (\"\")"), error in (no error)=w500) -> (VISA resource name out=w502:refnum<visa-resource-name>, error out=w501:errorcluster)  [unwired: 1 out]
        n142 = Concatenate Strings(w535, "-outputfpp-" ("Substring"), w536, w481, ".txt" ("Substring")) -> (w538:string)
        n143 = case shown="\"d\", Default" w525 {
          tunnel: [w550 w551] -> w523
          frame "s" {
            w550 = u16 0 items=["Single", "Double"] ("sweep mode")
          }
          frame "d", Default {
            w551 = u16 1 items=["Single", "Double"] ("sweep mode")
          }
        }
        n144 = Fract/Exp String To Number(string=w524) -> (number=w506:dbl[])  [unwired: 3 in, 1 out]
        n145 = String To Path(string=w538) -> (path=w534:path)
        n146 = Index Array(array=w506, index #1=0 ("Index")) -> (element #1=w522:dbl, element #2=w521:dbl, element #3=w520:dbl)  [unwired: 2 in]
        n147 = Delete From Array(array=w506, length=3 ("Length"), index=0 ("Index")) -> (array with subset deleted=w505:dbl[])  [unwired: 1 out]
        n148 = Bundle By Name(cluster=w514, "Gate Start"=w522, "Gate Stop"=w521, "Gate Step (linear only)"=w520, "Gate Compliance"=w532, "Range mode"=w498, "Range"=w497) -> (w548:T3)
        n149 = Index Array(array=w505, index #1=0 ("Index")) -> (element #1=w517:dbl, element #2=w516:dbl, element #3=w515:dbl)  [unwired: 2 in]
        n150 = call <vilib>:"compatOverwrite.vi"("overwrite (F)"=TRUE) -> ("overwrite?"=w486:T7)
        n151 = Bundle By Name(cluster=w513, "Drain Start"=w517, "Drain Stop"=w516, "Drain Step"=w515, "Drain Compliance"=w533, "Range mode"=w496, "Range"=w499) -> (w547:T4)
        n152 = call "4155C Output-FPP.vi"("VISA resource name in"=w502, "Gate"=w548, "Drain"=w547, "Timings"=w531, "error in (no error)"=w501, "sweep mode"=w523, "Panel controls"=w549) -> ("VD"=w491:dbl[], "Outparams"=w494:T8, "VISA Resource Name out"=w529:refnum<visa-resource-name>, "Vprobe2"=w490:dbl[], "ID"=w489:dbl[], "IG"=w488:dbl[], "Vprobe1"=w487:dbl[], "error out"=w530:errorcluster)  [unwired: 13 in]
        n153 = Unbundle By Name(w494) -> ("V2 Step"=w495:dbl, "V2 Start"=w493:dbl, "Number of points"=w492:i32)
        n154 = Open/Create/Replace File(file path (use dialog)=w534, error in=w530, operation (0:open)=w486) -> (refnum out=w544:refnum<file>, error out=w545:errorcluster)  [unwired: 3 in, 1 out]
        n155 = call "4155C Make Big 2d array FPP.vi"("1D Var1"=w491, "1d ID"=w489, "1d Vp2"=w490, "1d IG"=w488, "1d Vp1"=w487, "VAR2 START"=w493, "Number of VAR2 steps"=w492, "VAR2 STEP"=w495, "VAR1 Name"="Vd", "Decimal places in header"=i8 1, "VAR2 Name"="Vg") -> ("Header array"=w540:string[], "Data array"=w541:dbl[][])  [unwired: 15 in]
        n156 = call "4155C Write array to file.vi"("Byte Stream File Refnum"=w544, "Header"=w540, "Data Array"=w541, "error in (no error)"=w545) -> ("dup refnum"=w542:refnum<file>, "error out"=w543:errorcluster)  [unwired: 1 in]
        n157 = Close File(refnum=w542, error in=w543) -> (error out=w528:errorcluster)  [unwired: 1 out]
      }
      frame "itime" {
        n158 = Delete From Array(array=w565, index=0 ("Index")) -> (deleted portion=w566:string)  [unwired: 1 in, 1 out]
        n159 = case shown="\"l\"" w566 {
          tunnel: w564 -> [w570 w572 w575]
          tunnel: [w569 w571 w574] -> w557
          frame "s" {
            w568 = u32 0 items=["short  ", "medium  ", "long  "] ("integration time 2")
            n160 = Bundle By Name(cluster=w570, "integration time"=w568) -> (w569:T5)
          }
          frame "m", Default {
            w573 = u32 1 items=["short  ", "medium  ", "long  "] ("integration time 2")
            n161 = Bundle By Name(cluster=w572, "integration time"=w573) -> (w571:T5)
          }
          frame "l" {
            w576 = u32 2 items=["short  ", "medium  ", "long  "] ("integration time 2")
            n162 = Bundle By Name(cluster=w575, "integration time"=w576) -> (w574:T5)
          }
        }
      }
      frame "pulsed" {
        n163 = Delete From Array(array=w591, index=0 ("Index")) -> (deleted portion=w592:string, array with subset deleted=w579:string[])  [unwired: 1 in]
        n164 = case shown="\"on\", Default" w592 {
          tunnel: w590 -> [w602 w605]
          tunnel: [w601 w604] -> w583
          tunnel: w579 -> [w599 _]
          frame "on", Default {
            w600 = u16 1 items=["Continuous", "Pulsed"] ("sweep method")
            n165 = Fract/Exp String To Number(string=w599) -> (number=w597:dbl[])  [unwired: 3 in, 1 out]
            n166 = Index Array(array=w597, index #1=0 ("Index")) -> (element #1=w596:dbl, element #2=w595:dbl, element #3=w594:dbl)  [unwired: 2 in]
            n167 = Bundle By Name(cluster=w602, "sweep method"=w600, "Pulse period"=w596, "Base voltage"=w595, "Pulse width"=w594) -> (w601:T5)
          }
          frame "off" {
            w603 = u16 0 items=["Continuous", "Pulsed"] ("sweep method")
            n168 = Bundle By Name(cluster=w605, "sweep method"=w603) -> (w604:T5)
          }
        }
      }
      frame "gaterangemode" {
        n169 = Delete From Array(array=w618, index=0 ("Index")) -> (deleted portion=w619:string)  [unwired: 1 in, 1 out]
        n170 = case shown="\"f\"" w619 {
          tunnel: [w621 w622 w623] -> w608
          frame "a", Default {
            w621 = u16 0 items=["Auto", "Limited", "Fixed"] ("Gate Range\nmode 2")
          }
          frame "f" {
            w622 = u16 2 items=["Auto", "Limited", "Fixed"] ("Gate Range\nmode 2")
          }
          frame "l" {
            w623 = u16 1 items=["Auto", "Limited", "Fixed"] ("Gate Range\nmode 2")
          }
        }
      }
      frame "gaterange" {
        (unwired) u8 11 items=["10fA  ", "100fA  ", "1nA  ", "10nA", "100nA", "1uA", "10uA", "100uA", "1mA", "10mA", "100mA", "1A"] ("Gate Range 2")
        n171 = Delete From Array(array=w643, index=0 ("Index")) -> (deleted portion=w633:string)  [unwired: 1 in, 1 out]
        n172 = Scan Value(string=w633, format string="") -> (value=w631:dbl)  [unwired: 1 in, 1 out]
        n173 = Logarithm Base 10(1:w631) -> (0:w630:dbl)
        n174 = Round To Nearest(number=w630) -> (nearest integer value=w629:dbl)
        n175 = Add(x=w629, y=11.0) -> (x+y=w627:dbl)
        n176 = To Unsigned Byte Integer(number=w627) -> (unsigned 8bit integer=w626:u8)
      }
      frame "drainrange" {
        (unwired) u8 11 items=["10fA  ", "100fA  ", "1nA  ", "10nA", "100nA", "1uA", "10uA", "100uA", "1mA", "10mA", "100mA", "1A"] ("Gate Range 2")
        n177 = Delete From Array(array=w664, index=0 ("Index")) -> (deleted portion=w655:string)  [unwired: 1 in, 1 out]
        n178 = Scan Value(string=w655, format string="") -> (value=w653:dbl)  [unwired: 1 in, 1 out]
        n179 = Logarithm Base 10(1:w653) -> (0:w652:dbl)
        n180 = Round To Nearest(number=w652) -> (nearest integer value=w651:dbl)
        n181 = Add(x=w651, y=11.0) -> (x+y=w649:dbl)
        n182 = To Unsigned Byte Integer(number=w649) -> (unsigned 8bit integer=w648:u8)
      }
      frame "drainrangemode" {
        n183 = Delete From Array(array=w678, index=0 ("Index")) -> (deleted portion=w679:string)  [unwired: 1 in, 1 out]
        n184 = case shown="\"f\"" w679 {
          tunnel: [w681 w682 w683] -> w668
          frame "a", Default {
            w681 = u16 0 items=["Auto", "Limited", "Fixed"] ("Gate Range\nmode 2")
          }
          frame "f" {
            w682 = u16 2 items=["Auto", "Limited", "Fixed"] ("Gate Range\nmode 2")
          }
          frame "l" {
            w683 = u16 1 items=["Auto", "Limited", "Fixed"] ("Gate Range\nmode 2")
          }
        }
      }
      frame "Error", Default {
      }
      frame "logfile" {
        n185 = Number To Decimal String(number=w698) -> (decimal integer string=w733:string)  [unwired: 1 in]
        n186 = Concatenate Strings(w732, "logfile" ("Substring"), w733, w696, ".txt" ("Substring")) -> (w730:string)
        n187 = String To Path(string=w730) -> (path=w703:path)
        n188 = Unbundle(w729) -> ("integration time"=w728:u32, "Short/Long integration time"=w727:dbl, "hold time (sec)"=w726:dbl, "delay time (sec)"=w725:dbl, "Step Time (0 disables)"=w724:dbl, "sweep method"=w723:u16, "Pulse period"=w722:dbl, "Base voltage"=w721:dbl, "Pulse width"=w720:dbl)
        n189 = Build Array(w728, w727, w726, w725, w724, w723, w722, w721, w720, w714, w715, w716, w717, w718, w719) -> (w707:dbl[])
        n190 = Insert Into Array(array=dbl[][] [] ("Input Array"), new element=w707) -> (w706:dbl[][])  [unwired: 2 in]
        n191 = call <vilib>:"compatOverwrite.vi"("overwrite (F)"=TRUE) -> ("overwrite?"=w701:T7)
        n192 = Open/Create/Replace File(file path (use dialog)=w703, error in=w705, operation (0:open)=w701) -> (refnum out=w711:refnum<file>, error out=w710:errorcluster)  [unwired: 3 in, 1 out]
        n193 = call "4155C Write array to file.vi"("Byte Stream File Refnum"=w711, "Header"=string[] ["Int Time", "Short/Long Itime", "Hold time", "Delay time", "Step time", "Sweep method", "Pulse period", "Base Voltage", "Pulse width", "Drain compliance", "Gate compliance", "Gate range mode", "Gate range", "S/D range mode", "S/D range"], "Data Array"=w706, "error in (no error)"=w710) -> ("dup refnum"=w713:refnum<file>, "error out"=w712:errorcluster)  [unwired: 1 in]
        n194 = Close File(refnum=w713, error in=w712) -> (error out=w704:errorcluster)  [unwired: 1 out]
      }
      frame "sample" {
        n195 = Number To Decimal String(number=w737) -> (decimal integer string=w785:string)  [unwired: 1 in]
        n196 = Fract/Exp String To Number(string=w782) -> (number=w743:dbl[])  [unwired: 3 in, 1 out]
        n197 = Concatenate Strings(w760, "-sample-" ("Substring"), w785, w735, ".txt" ("Substring")) -> (w783:string)
        n198 = String To Path(string=w783) -> (path=w764:path)
        n199 = Index Array(array=w743, index=0 ("Index")) -> (element=w780:dbl)
        n200 = Index Array(array=w743, index=2 ("Index")) -> (element=w776:dbl)
        n201 = Index Array(array=w743, index=3 ("Index")) -> (element=w745:dbl)
        n202 = Index Array(array=w743, index=4 ("Index")) -> (element=w742:dbl)
        n203 = call "4155C Config Sampling Measurements.vi"("Sampling interval"=w742, "Sample time"=w745, "Display on/off"=TRUE, "Timings"=w751, "Num Points"=w776, "error in (no error)"=w787, "Drain Compliance"=w786, "Gate Compliance"=w761, "VISA session"=w788) -> ("error out"=w789:errorcluster, "dup VISA resource name"=w790:refnum<visa-resource-name>)  [unwired: 1 in]
        n204 = Index Array(array=w743, index=1 ("Index")) -> (element=w777:dbl)
        n205 = call "4155C Take Sample.vi"("Emergency Stop"=w757, "error in (no error)"=w789, "Vd"=w777, "Vg"=w780, "VISA resource name in"=w790) -> ("error out"=w755:errorcluster, "Id"=w792:dbl[], "Ig"=w766:dbl[], "VISA Resource Name out"=w753:refnum<visa-resource-name>, "Is"=w791:dbl[], "Time"=w770:dbl[])  [unwired: 1 in]
        n206 = Insert Into Array(array=dbl[][] [] ("Input Array"), new element=w770) -> (w769:dbl[][])  [unwired: 2 in]
        n207 = Insert Into Array(array=w769, new element=w766) -> (w768:dbl[][])  [unwired: 2 in]
        n208 = Insert Into Array(array=w768, new element=w792) -> (w767:dbl[][])  [unwired: 2 in]
        n209 = VISA Write(VISA resource name=w753, write buffer=":DISP ON" ("write buffer (\"\")"), error in (no error)=w755) -> (VISA resource name out=w752:refnum<visa-resource-name>, error out=w754:errorcluster)  [unwired: 1 out]
        n210 = Insert Into Array(array=w767, new element=w791) -> (w759:dbl[][])  [unwired: 2 in]
        n211 = Transpose 2D Array(2D array=w759) -> (transposed array=w758:dbl[][])
        n212 = call <vilib>:"compatOverwrite.vi"("overwrite (F)"=TRUE) -> ("overwrite?"=w740:T7)
        n213 = Open/Create/Replace File(file path (use dialog)=w764, error in=w754, operation (0:open)=w740) -> (refnum out=w773:refnum<file>, error out=w772:errorcluster)  [unwired: 3 in, 1 out]
        n214 = call "4155C Write array to file.vi"("Byte Stream File Refnum"=w773, "Header"=string[] ["Time /s", "Ig /A", "Id /A", "Is /A"], "Data Array"=w758, "error in (no error)"=w772) -> ("dup refnum"=w775:refnum<file>, "error out"=w774:errorcluster)  [unwired: 1 in]
        n215 = Close File(refnum=w775, error in=w774) -> (error out=w762:errorcluster)  [unwired: 1 out]
      }
      frame "samplei" {
        n216 = Number To Decimal String(number=w794) -> (decimal integer string=w846:string)  [unwired: 1 in]
        n217 = Fract/Exp String To Number(string=w843) -> (number=w810:dbl[])  [unwired: 3 in, 1 out]
        n218 = Concatenate Strings(w825, "-samplei-" ("Substring"), w846, w793, ".txt" ("Substring")) -> (w844:string)
        n219 = String To Path(string=w844) -> (path=w828:path)
        n220 = Index Array(array=w810, index=4 ("Index")) -> (element=w804:dbl)
        n221 = Index Array(array=w810, index=3 ("Index")) -> (element=w805:dbl)
        n222 = Index Array(array=w810, index=1 ("Index")) -> (element=w807:dbl)
        n223 = Index Array(array=w810, index=0 ("Index")) -> (element=w808:dbl)
        n224 = Index Array(array=w810, index=2 ("Index")) -> (element=w806:dbl)
        n225 = call "4155C Config SamplingI Measurements.vi"("Sample time"=w806, "Display on/off"=TRUE, "Timings"=w817, "Num Points"=w807, "error in (no error)"=w848, "Sampling interval"=w805, "VISA session"=w849) -> ("error out"=w850:errorcluster, "dup VISA resource name"=w851:refnum<visa-resource-name>)  [unwired: 3 in]
        n226 = call "4155C Take SampleI.vi"("Emergency Stop"=w822, "error in (no error)"=w850, "Idg 2"=w808, "Vdg compliance 2"=w804, "VISA resource name in"=w851) -> ("error out"=w820:errorcluster, "Idg"=w853:dbl[], "Vdg"=w830:dbl[], "VISA Resource Name out"=w818:refnum<visa-resource-name>, "Is"=w852:dbl[], "Time"=w834:dbl[])  [unwired: 1 in]
        n227 = Insert Into Array(array=dbl[][] [] ("Input Array"), new element=w834) -> (w833:dbl[][])  [unwired: 2 in]
        n228 = Insert Into Array(array=w833, new element=w830) -> (w832:dbl[][])  [unwired: 2 in]
        n229 = Insert Into Array(array=w832, new element=w853) -> (w831:dbl[][])  [unwired: 2 in]
        n230 = VISA Write(VISA resource name=w818, write buffer=":DISP ON" ("write buffer (\"\")"), error in (no error)=w820) -> (VISA resource name out=w803:refnum<visa-resource-name>, error out=w819:errorcluster)  [unwired: 1 out]
        n231 = Insert Into Array(array=w831, new element=w852) -> (w824:dbl[][])  [unwired: 2 in]
        n232 = Transpose 2D Array(2D array=w824) -> (transposed array=w823:dbl[][])
        n233 = call <vilib>:"compatOverwrite.vi"("overwrite (F)"=TRUE) -> ("overwrite?"=w798:T7)
        n234 = Open/Create/Replace File(file path (use dialog)=w828, error in=w819, operation (0:open)=w798) -> (refnum out=w837:refnum<file>, error out=w836:errorcluster)  [unwired: 3 in, 1 out]
        n235 = call "4155C Write array to file.vi"("Byte Stream File Refnum"=w837, "Header"=string[] ["Time /s", "Vdg /V", "Idg /A", "Is /A"], "Data Array"=w823, "error in (no error)"=w836) -> ("dup refnum"=w839:refnum<file>, "error out"=w838:errorcluster)  [unwired: 1 in]
        n236 = Close File(refnum=w839, error in=w838) -> (error out=w801:errorcluster)  [unwired: 1 out]
        n237 = VISA Write(VISA resource name=w803, write buffer=";:PAGE:SCON:STAN OFF;:PAGE:CHAN:VSU2:DIS;" ("write buffer (\"\")"), error in (no error)=w801) -> (VISA resource name out=w799:refnum<visa-resource-name>, error out=w800:errorcluster)  [unwired: 1 out]
      }
      frame "#" {
        n238 = VISA Write(VISA resource name=w860, write buffer=":DISP ON" ("write buffer (\"\")"), error in (no error)=w859) -> (VISA resource name out=w858:refnum<visa-resource-name>, error out=w857:errorcluster)  [unwired: 1 out]
      }
      frame "stressV" {
        n239 = Number To Decimal String(number=w870) -> (decimal integer string=w911:string)  [unwired: 1 in]
        n240 = Fract/Exp String To Number(string=w908) -> (number=w881:dbl[])  [unwired: 3 in, 1 out]
        n241 = Concatenate Strings(w895, "-stressV-" ("Substring"), w911, w869, ".txt" ("Substring")) -> (w909:string)
        n242 = String To Path(string=w909) -> (path=w899:path)
        n243 = Index Array(array=w881, index=3 ("Index")) -> (element=w878:dbl)
        n244 = Index Array(array=w881, index=1 ("Index")) -> (element=w876:dbl)
        n245 = Index Array(array=w881, index=0 ("Index")) -> (element=w875:dbl)
        n246 = Index Array(array=w881, index=4 ("Index")) -> (element=w880:dbl)
        n247 = Index Array(array=w881, index=2 ("Index")) -> (element=w877:dbl)
        n248 = call "4155C Config V Stress.vi"("VISA session"=w914, "ID compliance"=w878, "VD"=w876, "VG"=w875, "IG compliance"=w877, "error in (no error)"=w913, "Display on/off"=TRUE) -> ("dup VISA resource name"=w916:refnum<visa-resource-name>, "error out"=w915:errorcluster)
        n249 = call "4155C Apply Stress.vi"("error in (no error)"=w915, "Duration"=w880, "Emergency Stop"=w894, "VISA resource name in"=w916) -> ("error out"=w892:errorcluster, "VISA Resource Name out"=w890:refnum<visa-resource-name>)
        n250 = VISA Write(VISA resource name=w890, write buffer=":DISP ON" ("write buffer (\"\")"), error in (no error)=w892) -> (VISA resource name out=w889:refnum<visa-resource-name>, error out=w891:errorcluster)  [unwired: 1 out]
        n251 = call <vilib>:"compatOverwrite.vi"("overwrite (F)"=TRUE) -> ("overwrite?"=w874:T7)
        n252 = Open/Create/Replace File(file path (use dialog)=w899, error in=w891, operation (0:open)=w874) -> (refnum out=w902:refnum<file>, error out=w901:errorcluster)  [unwired: 3 in, 1 out]
        n253 = call "4155C Write array to file.vi"("Byte Stream File Refnum"=w902, "Header"=string[] ["V stress completed successfully", ""], "error in (no error)"=w901) -> ("dup refnum"=w904:refnum<file>, "error out"=w903:errorcluster)  [unwired: 2 in]
        n254 = Close File(refnum=w904, error in=w903) -> (error out=w897:errorcluster)  [unwired: 1 out]
      }
      frame "stressI" {
        n255 = Number To Decimal String(number=w918) -> (decimal integer string=w955:string)  [unwired: 1 in]
        n256 = Fract/Exp String To Number(string=w952) -> (number=w927:dbl[])  [unwired: 3 in, 1 out]
        n257 = Concatenate Strings(w939, "-stressI-" ("Substring"), w955, w917, ".txt" ("Substring")) -> (w953:string)
        n258 = String To Path(string=w953) -> (path=w943:path)
        n259 = Index Array(array=w927, index=1 ("Index")) -> (element=w923:dbl)
        n260 = Index Array(array=w927, index=0 ("Index")) -> (element=w924:dbl)
        n261 = call "4155C Config I Stress.vi"("VISA session"=w958, "IDG"=w924, "VDG compliance"=w923, "error in (no error)"=w957, "Display on/off"=TRUE) -> ("dup VISA resource name"=w960:refnum<visa-resource-name>, "error out"=w959:errorcluster)
        n262 = Index Array(array=w927, index=2 ("Index")) -> (element=w925:dbl)
        n263 = call "4155C Apply Stress.vi"("error in (no error)"=w959, "Duration"=w925, "Emergency Stop"=w938, "VISA resource name in"=w960) -> ("error out"=w936:errorcluster, "VISA Resource Name out"=w934:refnum<visa-resource-name>)
        n264 = VISA Write(VISA resource name=w934, write buffer=":DISP ON" ("write buffer (\"\")"), error in (no error)=w936) -> (VISA resource name out=w933:refnum<visa-resource-name>, error out=w935:errorcluster)  [unwired: 1 out]
        n265 = call <vilib>:"compatOverwrite.vi"("overwrite (F)"=TRUE) -> ("overwrite?"=w922:T7)
        n266 = Open/Create/Replace File(file path (use dialog)=w943, error in=w935, operation (0:open)=w922) -> (refnum out=w946:refnum<file>, error out=w945:errorcluster)  [unwired: 3 in, 1 out]
        n267 = call "4155C Write array to file.vi"("Byte Stream File Refnum"=w946, "Header"=string[] ["I stress completed successfully", ""], "error in (no error)"=w945) -> ("dup refnum"=w948:refnum<file>, "error out"=w947:errorcluster)  [unwired: 2 in]
        n268 = Close File(refnum=w948, error in=w947) -> (error out=w941:errorcluster)  [unwired: 1 out]
      }
      frame "vsu2pulse" {
        n269 = Number To Decimal String(number=w962) -> (decimal integer string=w997:string)  [unwired: 1 in]
        n270 = Fract/Exp String To Number(string=w994) -> (number=w970:dbl[])  [unwired: 3 in, 1 out]
        n271 = Concatenate Strings(w982, "-vsu2-" ("Substring"), w997, w961, ".txt" ("Substring")) -> (w995:string)
        n272 = String To Path(string=w995) -> (path=w986:path)
        n273 = Index Array(array=w970, index=1 ("Index")) -> (element=w969:dbl)
        n274 = Index Array(array=w970, index=0 ("Index")) -> (element=w967:dbl)
        n275 = call "4155C Config VSU2 Stress.vi"("error in (no error)"=w999, "VSU2"=w967, "Display on/off"=TRUE, "VISA session"=w1000) -> ("error out"=w1001:errorcluster, "dup VISA resource name"=w1002:refnum<visa-resource-name>)
        n276 = call "4155C Apply Stress.vi"("error in (no error)"=w1001, "Duration"=w969, "Emergency Stop"=w981, "VISA resource name in"=w1002) -> ("error out"=w979:errorcluster, "VISA Resource Name out"=w977:refnum<visa-resource-name>)
        n277 = VISA Write(VISA resource name=w977, write buffer=":DISP ON" ("write buffer (\"\")"), error in (no error)=w979) -> (VISA resource name out=w976:refnum<visa-resource-name>, error out=w978:errorcluster)  [unwired: 1 out]
        n278 = call <vilib>:"compatOverwrite.vi"("overwrite (F)"=TRUE) -> ("overwrite?"=w966:T7)
        n279 = Open/Create/Replace File(file path (use dialog)=w986, error in=w978, operation (0:open)=w966) -> (refnum out=w989:refnum<file>, error out=w988:errorcluster)  [unwired: 3 in, 1 out]
        n280 = call "4155C Write array to file.vi"("Byte Stream File Refnum"=w989, "Header"=string[] ["VSU2 pulse completed successfully", ""], "error in (no error)"=w988) -> ("dup refnum"=w991:refnum<file>, "error out"=w990:errorcluster)  [unwired: 2 in]
        n281 = Close File(refnum=w991, error in=w990) -> (error out=w984:errorcluster)  [unwired: 1 out]
      }
      frame "sample-fpp" {
        w1015 = string[] ["Time /s", "Id VgVd /A", "Ig VgVd /A", "Vp1 VgVd /V", "Vp2 VgVd /V"] ("Header")
        w1019 = "%d" ("format string")
        n282 = Number To Decimal String(number=w1004) -> (decimal integer string=w1067:string)  [unwired: 1 in]
        n283 = Fract/Exp String To Number(string=w1064) -> (number=w1052:dbl[])  [unwired: 3 in, 1 out]
        n284 = Concatenate Strings(w1058, "-samplefpp-" ("Substring"), w1067, w1003, ".txt" ("Substring")) -> (w1065:string)
        n285 = String To Path(string=w1065) -> (path=w1027:path)
        n286 = Index Array(array=w1052, index=0 ("Index")) -> (element=w1013:dbl)
        n287 = Index Array(array=w1052, index=1 ("Index")) -> (element=w1012:dbl)
        n288 = Index Array(array=w1052, index=2 ("Index")) -> (element=w1060:dbl)
        n289 = Index Array(array=w1052, index=3 ("Index")) -> (element=w1050:dbl)
        n290 = call "4155C Config Sampling Measurements FPP.vi"("VISA session"=w1070, "Num Points"=w1060, "Vg"=w1013, "Display on/off"=TRUE, "Gate Compliance"=w1059, "Drain Compliance"=w1068, "Standby"="Standby", "error in (no error)"=w1069, "Timings"=w1057, "Vd"=w1012, "Sample time"=w1050) -> ("dup VISA resource name"=w1029:refnum<visa-resource-name>, "error out"=w1028:errorcluster)  [unwired: 3 in]
        n291 = Number To Decimal String(number=w1013) -> (decimal integer string=w1039:string)  [unwired: 1 in]
        n292 = call "4155C Take Sample FPP.vi"("VISA resource name in"=w1029, "error in (no error)"=w1028, "Emergency Stop"=w1030) -> ("Time"=w1034:dbl[], "Vp1"=w1044:dbl[], "VISA Resource Name out"=w1010:refnum<visa-resource-name>, "Ig"=w1032:dbl[], "Id"=w1033:dbl[], "Vp2"=w1042:dbl[], "error out"=w1031:errorcluster)  [unwired: 10 in]
        n293 = Insert Into Array(array=dbl[][] [] ("Input Array"), new element=w1034) -> (w1048:dbl[][])  [unwired: 2 in]
        n294 = Number To Decimal String(number=w1012) -> (decimal integer string=w1037:string)  [unwired: 1 in]
        n295 = Insert Into Array(array=w1048, new element=w1033) -> (w1047:dbl[][])  [unwired: 2 in]
        n296 = Concatenate Strings("(Vg = " ("Substring"), w1039, "V, Vd = " ("Substring"), w1037, "V)" ("Substring")) -> (w1035:string)
        n297 = Insert Into Array(array=w1047, new element=w1032) -> (w1046:dbl[][])  [unwired: 2 in]
        n298 = Insert Into Array(array=w1046, new element=w1044) -> (w1043:dbl[][])  [unwired: 2 in]
        n299 = Insert Into Array(array=w1043, new element=w1042) -> (w1011:dbl[][])  [unwired: 2 in]
        n300 = call <vilib>:"compatOverwrite.vi"("overwrite (F)"=TRUE) -> ("overwrite?"=w1008:T7)
        n301 = Open/Create/Replace File(file path (use dialog)=w1027, error in=w1031, operation (0:open)=w1008) -> (refnum out=w1024:refnum<file>, error out=w1025:errorcluster)  [unwired: 3 in, 1 out]
        n302 = Array To Spreadsheet String(array=w1015, 3:w1019) -> (spreadsheet string=w1021:string)  [unwired: 1 in]
        n303 = Transpose 2D Array(2D array=w1011) -> (transposed array=w1041:dbl[][])
        n304 = Search and Replace String(replace all?=TRUE ("replace all? (F)"), input string=w1021, search string="VgVd", replace string=w1035) -> (result string=w1017:string)  [unwired: 4 in, 3 out]
        n305 = Spreadsheet String To Array(format string=w1019, spreadsheet string=w1017, array type (2D Dbl)=w1015) -> (array=w1016:string[])  [unwired: 1 in]
        n306 = call "4155C Write array to file.vi"("Byte Stream File Refnum"=w1024, "Header"=w1016, "Data Array"=w1041, "error in (no error)"=w1025) -> ("dup refnum"=w1022:refnum<file>, "error out"=w1023:errorcluster)  [unwired: 1 in]
        n307 = Close File(refnum=w1022, error in=w1023) -> (error out=w1009:errorcluster)  [unwired: 1 out]
      }
      frame "resample-fpp" {
        w1085 = string[] ["Time /s", "Id VgVd /A", "Ig VgVd /A", "Vp1 VgVd /V", "Vp2 VgVd /V"] ("Header")
        w1089 = "%d" ("format string")
        n308 = Number To Decimal String(number=w1071) -> (decimal integer string=w1129:string)  [unwired: 1 in]
        n309 = Fract/Exp String To Number(string=w1126) -> (number=w1078:dbl[])  [unwired: 3 in, 1 out]
        n310 = Concatenate Strings(w1122, "-resamplefpp-" ("Substring"), w1129, w1072, ".txt" ("Substring")) -> (w1127:string)
        n311 = String To Path(string=w1127) -> (path=w1097:path)
        n312 = Index Array(array=w1078, index=0 ("Index")) -> (element=w1084:dbl)
        n313 = Index Array(array=w1078, index=1 ("Index")) -> (element=w1083:dbl)
        n314 = Number To Decimal String(number=w1084) -> (decimal integer string=w1107:string)  [unwired: 1 in]
        n315 = call "4155C Take Sample FPP.vi"("VISA resource name in"=w1080, "error in (no error)"=w1079, "Emergency Stop"=w1098) -> ("Time"=w1102:dbl[], "Vp1"=w1112:dbl[], "VISA Resource Name out"=w1082:refnum<visa-resource-name>, "Ig"=w1100:dbl[], "Id"=w1101:dbl[], "Vp2"=w1110:dbl[], "error out"=w1099:errorcluster)  [unwired: 10 in]
        n316 = Insert Into Array(array=dbl[][] [] ("Input Array"), new element=w1102) -> (w1116:dbl[][])  [unwired: 2 in]
        n317 = Number To Decimal String(number=w1083) -> (decimal integer string=w1105:string)  [unwired: 1 in]
        n318 = Insert Into Array(array=w1116, new element=w1101) -> (w1115:dbl[][])  [unwired: 2 in]
        n319 = Concatenate Strings("(Vg = " ("Substring"), w1107, "V, Vd = " ("Substring"), w1105, "V)" ("Substring")) -> (w1103:string)
        n320 = Insert Into Array(array=w1115, new element=w1100) -> (w1114:dbl[][])  [unwired: 2 in]
        n321 = Insert Into Array(array=w1114, new element=w1112) -> (w1111:dbl[][])  [unwired: 2 in]
        n322 = Insert Into Array(array=w1111, new element=w1110) -> (w1077:dbl[][])  [unwired: 2 in]
        n323 = call <vilib>:"compatOverwrite.vi"("overwrite (F)"=TRUE) -> ("overwrite?"=w1076:T7)
        n324 = Open/Create/Replace File(file path (use dialog)=w1097, error in=w1099, operation (0:open)=w1076) -> (refnum out=w1094:refnum<file>, error out=w1095:errorcluster)  [unwired: 3 in, 1 out]
        n325 = Array To Spreadsheet String(array=w1085, 3:w1089) -> (spreadsheet string=w1091:string)  [unwired: 1 in]
        n326 = Transpose 2D Array(2D array=w1077) -> (transposed array=w1109:dbl[][])
        n327 = Search and Replace String(replace all?=TRUE ("replace all? (F)"), input string=w1091, search string="VgVd", replace string=w1103) -> (result string=w1087:string)  [unwired: 4 in, 3 out]
        n328 = Spreadsheet String To Array(format string=w1089, spreadsheet string=w1087, array type (2D Dbl)=w1085) -> (array=w1086:string[])  [unwired: 1 in]
        n329 = call "4155C Write array to file.vi"("Byte Stream File Refnum"=w1094, "Header"=w1086, "Data Array"=w1109, "error in (no error)"=w1095) -> ("dup refnum"=w1092:refnum<file>, "error out"=w1093:errorcluster)  [unwired: 1 in]
        n330 = Close File(refnum=w1092, error in=w1093) -> (error out=w1081:errorcluster)  [unwired: 1 out]
      }
      frame "serial" {
        n331 = Index Array(array=w1133, index=0 ("Index")) -> (element=w1132:string)
        n332 = call "Serial write and read v0.4.vi"("Termination char\n(0xA = '\\n' = LF)\n(0xD = '\\r' = CR)"="Termination char\n(0xA = '\\n' = LF)\n(0xD = '\\r' = CR)", "Enable Termination\nChar (T)"="Enable Termination\nChar (T)", "parity"="parity", "stop bits"="stop bits", "string to write"=w1132, "flow control"="flow control", "byte count"="byte count", "Serial Settings:Serial End Mode for Reads"="Serial Settings:Serial End Mode for Reads", "Timeout (ms)"="Timeout (ms)", "error in (no error)"=w1138, "VISA resource name"="VISA resource name", "baud rate"="baud rate", "data bits"="data bits") -> ("read string"=→"Serial port output":string, "error out"=w1137:errorcluster)  [unwired: 1 in]
      }
    }
    n333 = Build Array("Time /s" ("element"), "Id max /A" ("VAR2 Name")) -> (w59:string[])
    n334 = Build Array(w54, w53) -> (w52:dbl[][])
    n335 = Transpose 2D Array(2D array=w52) -> (transposed array=w51:dbl[][])
    n336 = Concatenate Strings(w50, "-Ion-", ".txt" ("Suffix")) -> (w67:string)
    n337 = Array To Spreadsheet String(array=w59, 3:"" ("format string")) -> (spreadsheet string=w58:string)  [unwired: 1 in]
    n338 = Array To Spreadsheet String(array=w51, 3:"%e" ("format string")) -> (spreadsheet string=w57:string)  [unwired: 1 in]
    n339 = String To Path(string=w67) -> (path=w66:path)
    n340 = Build Array(w58, w57) -> (w56:string[])
    n341 = Write to Text File(file (use dialog)=w66, text=w56, error in=w46) -> (refnum out=w68:refnum<file>, error out=w55:errorcluster)  [unwired: 1 in, 1 out]
    n342 = Close File(refnum=w68, error in=w55) -> (error out=w45:errorcluster)  [unwired: 1 out]
    "Line running" <- w78
    "Total lines" <- w77
  }
  "error out" <- w1
